vi "SPIM Controller.vi"() -> ()   [LabVIEW 2015]
uses:
  controls/Camera Properties.ctl
  controls/Microscope Settings.ctl
  controls/CameraState.ctl
  controls/ModeEnum.ctl
  controls/PinOut.ctl
  controls/Hardware.ctl
  controls/PinOut2.ctl
  controls/Stack_State.ctl
  controls/Stack Track.ctl
  controls/CameraControlTypeDef.ctl
  <vilib>/DAQmx/create/channels.llb/DAQmx Create Channel (DO-Digital Output).vi
  <vilib>/DAQmx/create/channels.llb/DAQmx Create Channel (AO-Voltage-Basic).vi
  <vilib>/Waveform/DWDTOps.llb/DWDT Append Digital Samples.vi
  <vilib>/Waveform/WDTOps.llb/WDT Append Waveforms DBL.vi
  <vilib>/Waveform/WDTOps.llb/WDT Waveform Duration DBL.vi
  <vilib>/vision/NI_Vision_Development_Module.lvlib
panel:
  out "Numeric 3":i32
  out "Numeric 2":i32
  out "Stack Number":i32
  out "Numeric":i32
  in  "Tab Control":enum32{"Camera Settings", "Recording"}(tab)
  in  "Scan Cont":bool
  in  "Tweezers":T1={"Start /um"=40.0, "Step/um"=5.0, "Range /um"=20.0} {"Range /um" min=0.0 max=10.0 step=0.05; "Step/um" min=0.0001 max=10.0 step=0.05; "Start /um" min=0.0 max=10.0 step=0.05}
  in  "Save to:":path=path "C:/_DATA/test.tiff"
  in  "Scans":dbl=1.0 min=0.0 max=10.0 step=0.05
  in  "?":bool
  in  "Scan":bool
  in  "Scan Continuously":bool
  out "error IO":errorcluster
  in  "Advanced DCAM Controls":i32(listbox) caption="Multicolumn Listbox"
  out "Duration":string
  in  "Microscope Settings":T2={"Mode"=enum."XY", "Slit"={"Scanning Mode"=12.0, "Slit Width /%"=5.0}, "Colour"=[{"Laser"=enum."561", "Filter"=4}], "Exposure/ms"=40.0, "Piezo Position /um"=0.0, "ROI"={"X"={"Start /px"=0.0, "Step /px"=1.0, "Range /px"=2048.0}, "Y"={"Start /px"=0.0, "Step /px"=1.0, "Range /px"=2048.0}, "Z "={"Start /um"=0.0, "Step/um"=1.0, "Range /um"=100.0}, "T "={"Start /s"=0.0, "Step /s"=1.0, "Range /s"=100.0}}, "Samples per millisecond"=100.0, "Relax/ms"=10.0, "Readout Direction"=2.0, "Trigger Source"=2.0, "Camera Delay /ms"=11.0, "Under Scan /ms"=5.0, "Calibration Coordinates"={"Top Left"=[-4.418670520231216, -0.1592138728323702, 10.0], "Top Right"=[-9.501965317919073, -0.1592138728323702, 10.0], "Bottom Left"=[-4.4508670520231215, 0.0, 0.0], "Bottom Right"=[-9.53757225433526, 0.0, 0.0], "Waveforms"={"Analogue Out"=[], "Digital Out"=[]}}} {"Under Scan /ms" min=0.0 max=10.0 step=0.05; "ROI"."T"."Range /s" min=0.0 max=10.0 step=0.05 format="%<%H:%M:%S>t"; "ROI"."T"."Step /s" min=0.0 max=10.0 step=0.05 format="%<%M:%S%2u>t"; "ROI"."T"."Start /s" min=0.0 max=10.0 step=0.05 format="%<%M:%S%2u>t"; "ROI"."X"."Range /px" min=0.0 max=10.0 step=0.05; "ROI"."X"."Step /px" min=0.0 max=10.0 step=0.05; "ROI"."X"."Start /px" min=0.0 max=10.0 step=0.05; "ROI"."Y"."Range /px" min=0.0 max=10.0 step=0.05; "ROI"."Y"."Step /px" min=0.0 max=10.0 step=0.05; "ROI"."Y"."Start /px" min=0.0 max=10.0 step=0.05; "ROI"."Z"."Range /um" min=0.0 max=10.0 step=0.05; "ROI"."Z"."Step/um" min=0.0001 max=10.0 step=0.05; "ROI"."Z"."Start /um" min=0.0 max=10.0 step=0.05; "Colour"."Filter" items=["Empty"=1, ""=2, ""=3, "561"=4, ""=5, "488"=6]; "Camera Delay /ms" min=0.0 max=10.0 step=0.05; "Trigger Source" items=["Internal"=1.0, "External"=2.0]; "Readout Direction" items=["Forward"=1.0, "Backward"=2.0]; "Slit"."Scanning Mode" items=["Full Frame"=1.0, "Slit Scanning"=12.0]; "Piezo Position /um" min=0.0 max=10.0 step=0.05}
  in  "Properties":T3=4211904 items=["SENSOR MODE"=4212128, "CCD MODE"=4212384, "READOUT MODE"=4211872, "ACTIVE VIEW INDEX"=4343136, "BITS PER CHANNEL"=4342976, "IMAGE PIXEL TYPE"=4343296, "BINNING"=4215968, "EXPOSURE TIME"=2049184, "CONTRAST GAIN"=3163312, "CONTRAST OFFSET"=3163328, "LIGHT MODE"=2114720, "SENSITIVITY"=2114992, "PHOTON IMAGING MODE"=2115200, "HIGH DYNAMIC RANGE MODE"=3163360, "WHITE BALANCE"=3163568, "TEMPERATURE"=2115232, "TEMPERATURE TARGET"=2115264, "SENSOR COOLER FAN"=2115296, "LINEBUNDLE HEIGHT"=4212192, "MECHANICAL SHUTTER"=2115488, "BACK FOCUS POSITION"=8422304, "TRIGGER CONNECTOR"=1066432, "TRIGGER SOURCE"=1066144, "OUTPUT TRIGGER SOURCE"=1852576, "TRIGGER GLOBAL EXPOSURE"=2049680, "FIRST TRIGGER BEHAVIOR"=2049696, "CHANNEL SYNC"=1852352, "READOUT DIRECTION"=4211904, "PRE HSYNC COUNT"=1852704, "INTERNAL LINE SPEED"=4191408, "INTERNAL LINE INVERVAL"=4191424]
  out "Enum":T4=enum."active"
  out "FPS":dbl
  in  "Multicolumn Listbox":i32(listbox)
  out "Image":T5(plugin-control)
  out "Histogram":T6(graph)
  in  "stop":bool
  in  "Load Settings":bool
  in  "Save Settings":bool
  in  "Frames":i32
  in  "Record":bool
  in  "Signals Debugger":bool
  in  "Stage Controller":bool
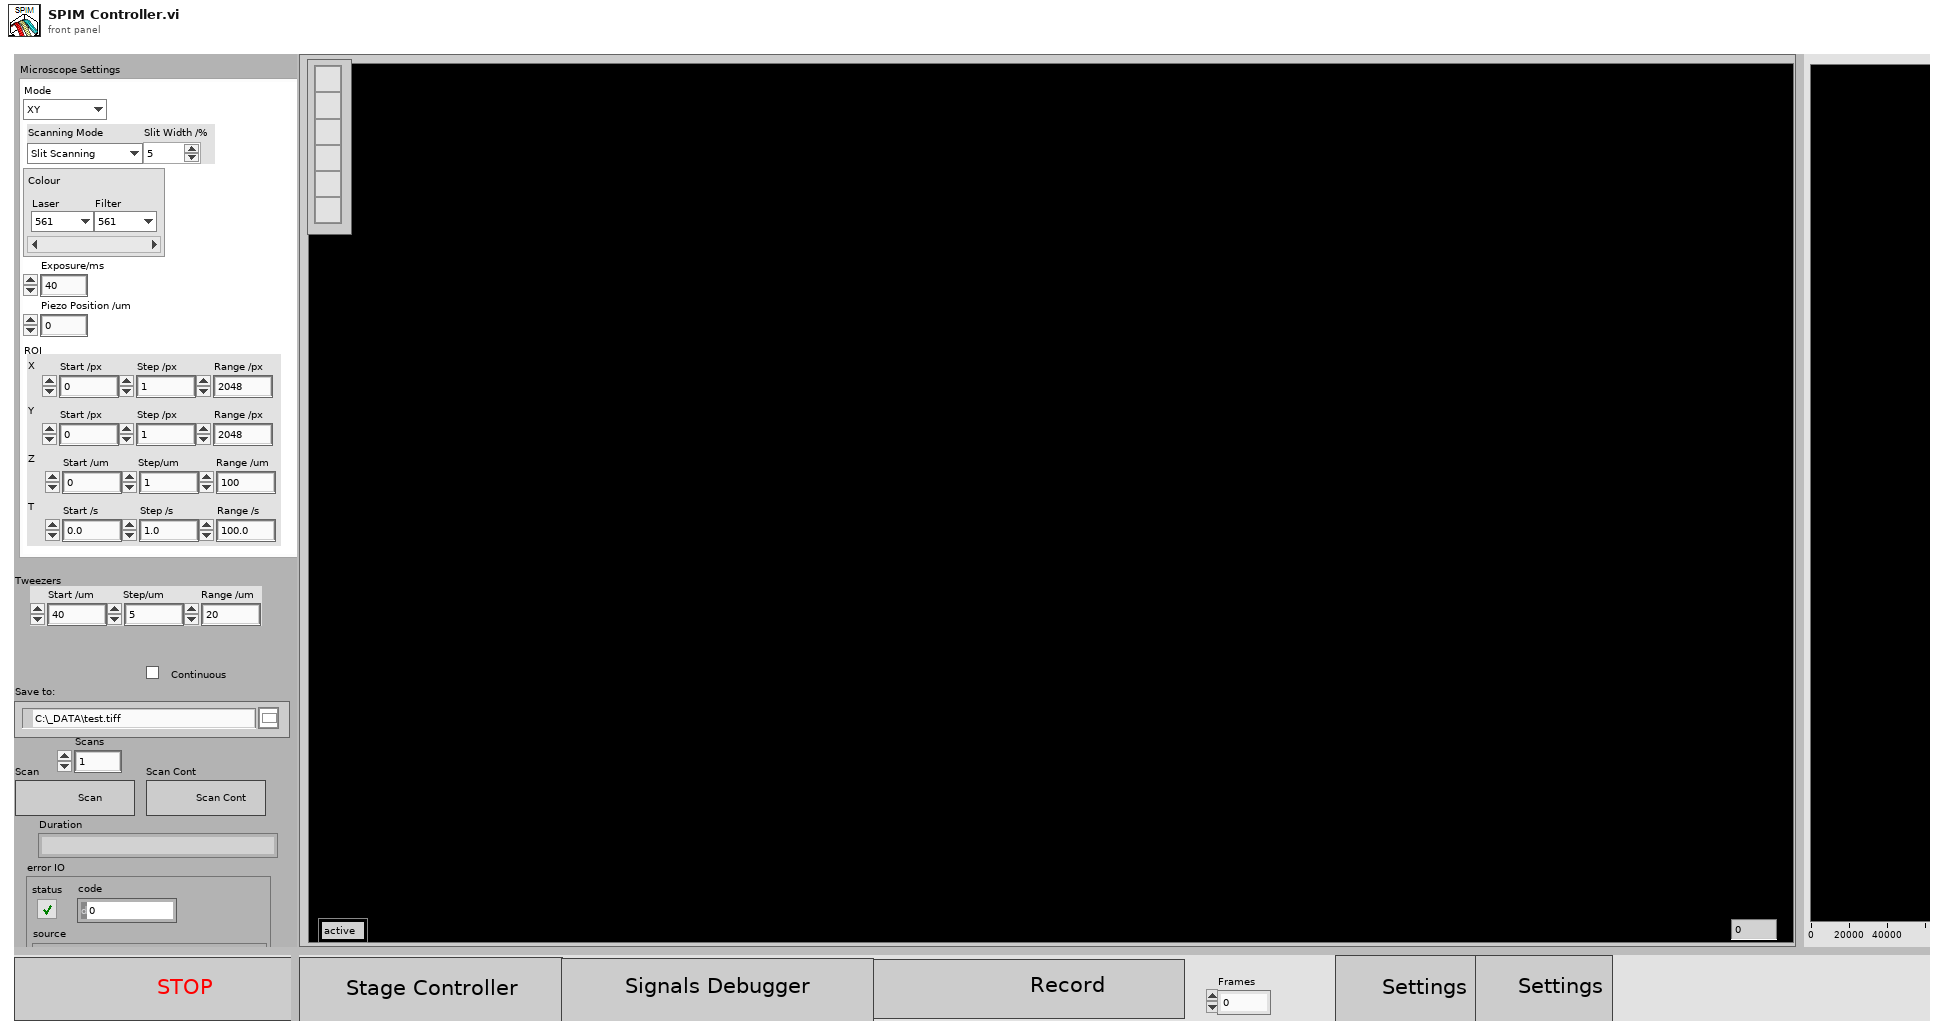
[diagram p1: front panel]
types:
  T1 = cluster{"Start /um":dbl, "Step/um":dbl, "Range /um":dbl}
  T2 = typedef "Microscope Settings.ctl" = cluster{"Mode":enum16{"X", "XY", "XYZ", "XYZT", "XYZC", "Tweezers", "Virus"}, "Slit":cluster{"Scanning Mode":dbl, "Slit Width /%":dbl}, "Colour":cluster{"Laser":enum16{"Brightfield", "445", "488", "561", "647"}, "Filter":u16}[], "Exposure/ms":dbl, "Piezo Position /um":dbl, "ROI":cluster{"X":cluster{"Start /px":dbl, "Step /px":dbl, "Range /px":dbl}, "Y":cluster{"Start /px":dbl, "Step /px":dbl, "Range /px":dbl}, "Z ":cluster{"Start /um":dbl, "Step/um":dbl, "Range /um":dbl}, "T ":cluster{"Start /s":dbl, "Step /s":dbl, "Range /s":dbl}}, "Samples per millisecond":dbl, "Relax/ms":dbl, "Readout Direction":dbl, "Trigger Source":dbl, "Camera Delay /ms":dbl, "Under Scan /ms":dbl, "Calibration Coordinates":cluster{"Top Left":dbl[], "Top Right":dbl[], "Bottom Left":dbl[], "Bottom Right":dbl[], "Waveforms":cluster{"Analogue Out":waveform(dbl)[], "Digital Out":digitalwaveform[]}}}
  T3 = typedef "Camera Properties.ctl" = u32
  T4 = typedef "CameraState.ctl" = enum16{"init", "active", "deinit"}
  T5 = typedef "IMAQ Image.ctl" = refnum<image>
  T6 = cluster{"Starting Value":sgl, "Incremental Value":sgl, "Histogram":u32[]}
  T7 = cluster{"height":u32, "width":u32, "datatype":u32}
  T8 = typedef "Hardware.ctl" = enum16{"Stop", "RunCont", "EndCont", "Idle", "Update", "Run Waves"}
  T9 = typedef "PinOut.ctl" = string
  T10 = typedef "ModeEnum.ctl" = enum16{"Idle", "generateWaves", "runWaves", "runWavesCont", "endWavesCont", "stop"}
  T11 = cluster{"Mode":u32, "Polarity":u32, "Times":u32, "Delay":dbl}
  T12 = typedef "Stack_State.ctl" = cluster{"State":T13, "Stack Number":i32, "Image":u16[][], "Stacks":i32}
  T13 = typedef "Stack Track.ctl" = enum16{"Idle", "Display", "Start Sequence", "Read Disk", "STOP", "Collecting", "End", "Save Image"}
  T14 = typedef "CameraControlTypeDef.ctl" = enum16{"Idle", "IntervalLineInt", "Ram Record", "HardDisk Record", "Disengage Update", "Update", "ROI", "Binning", "Scan Mode", "Trigger Mode", "Readout Mode", "Readout Direction", "Preview", "ROIWindow", "Trigger Source"}
  T15 = cluster{"Laser":enum16{"Brightfield", "445", "488", "561", "647"}, "Filter":u16}[]
  T16 = enum32{"Invalid", "Standard", "Closed", "Hidden", "Minimized", "Maximized"}
  T17 = enum16{"open", "replace", "create", "open or create", "replace or create", "replace or create with confirmation"}
  T18 = typedef "PinOut2.ctl" = string
  T19 = cluster{"Analogue Out":waveform(dbl)[], "Digital Out":digitalwaveform[]}
  T20 = enum16{"X", "XY", "XYZ", "XYZT", "XYZC", "Tweezers", "Virus"}
  T21 = typedef "Image Type" = u32
  T22 = cluster{"Analogue Out out":waveform(dbl)[], "Digital Out out":digitalwaveform[]}
  T23 = cluster{"State":T13, "Timeout":i32, "Data 16":u16[][], "Timeout":i32}
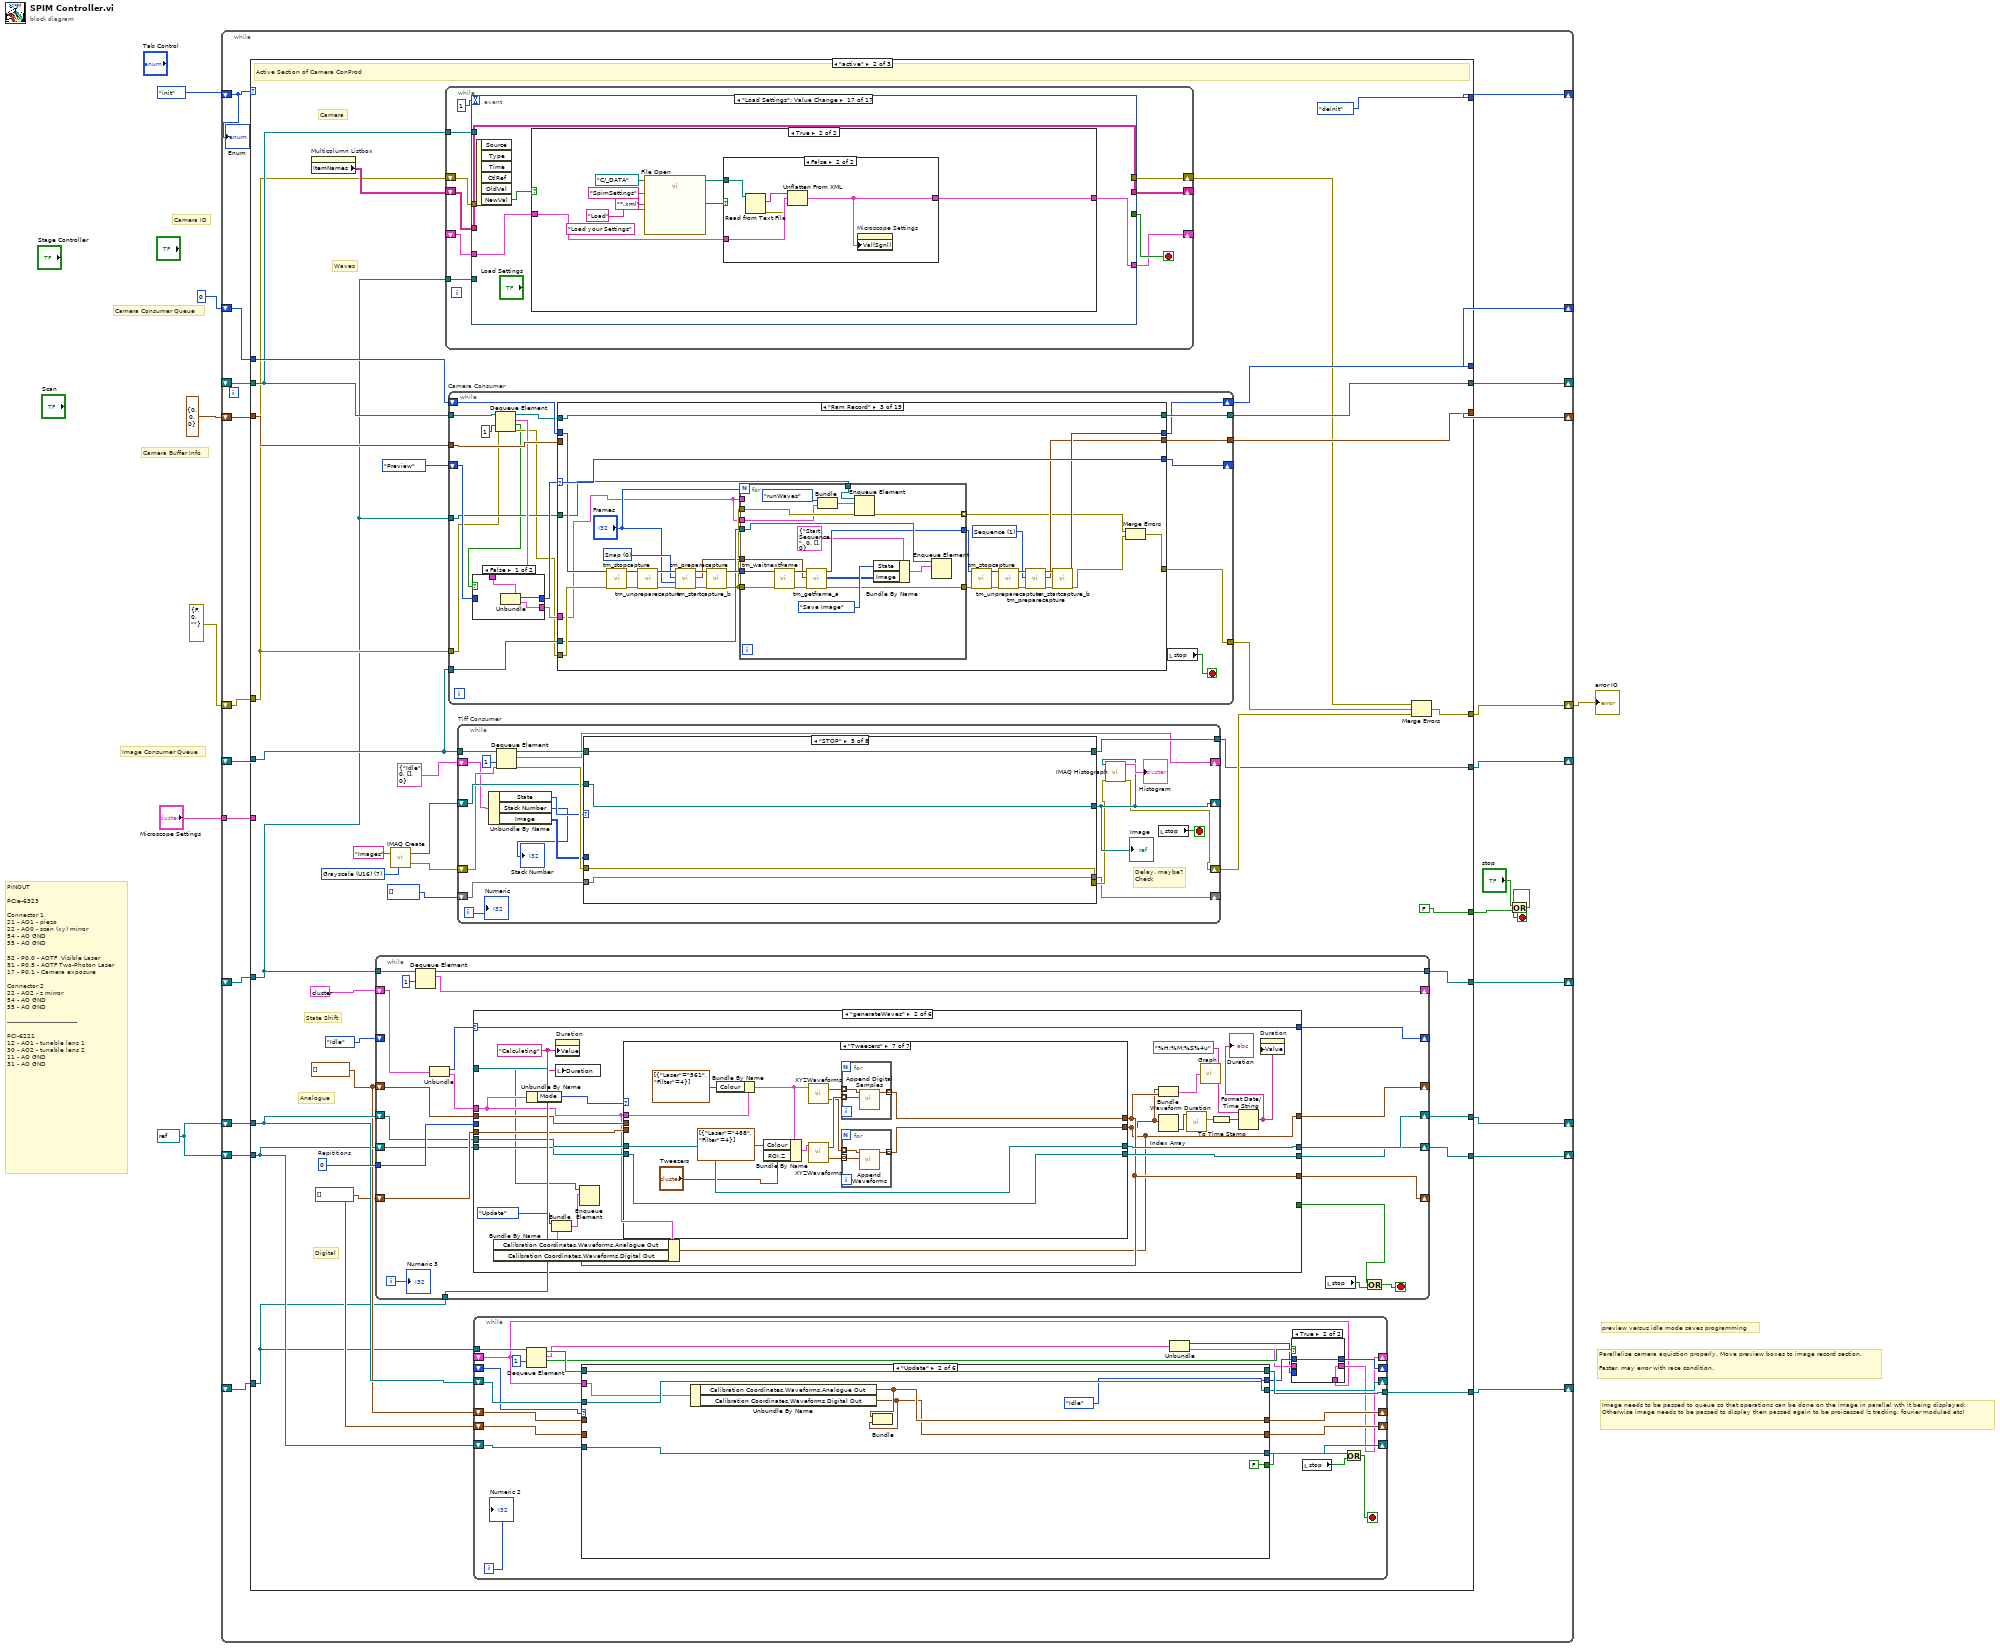
[diagram p0: block diagram]
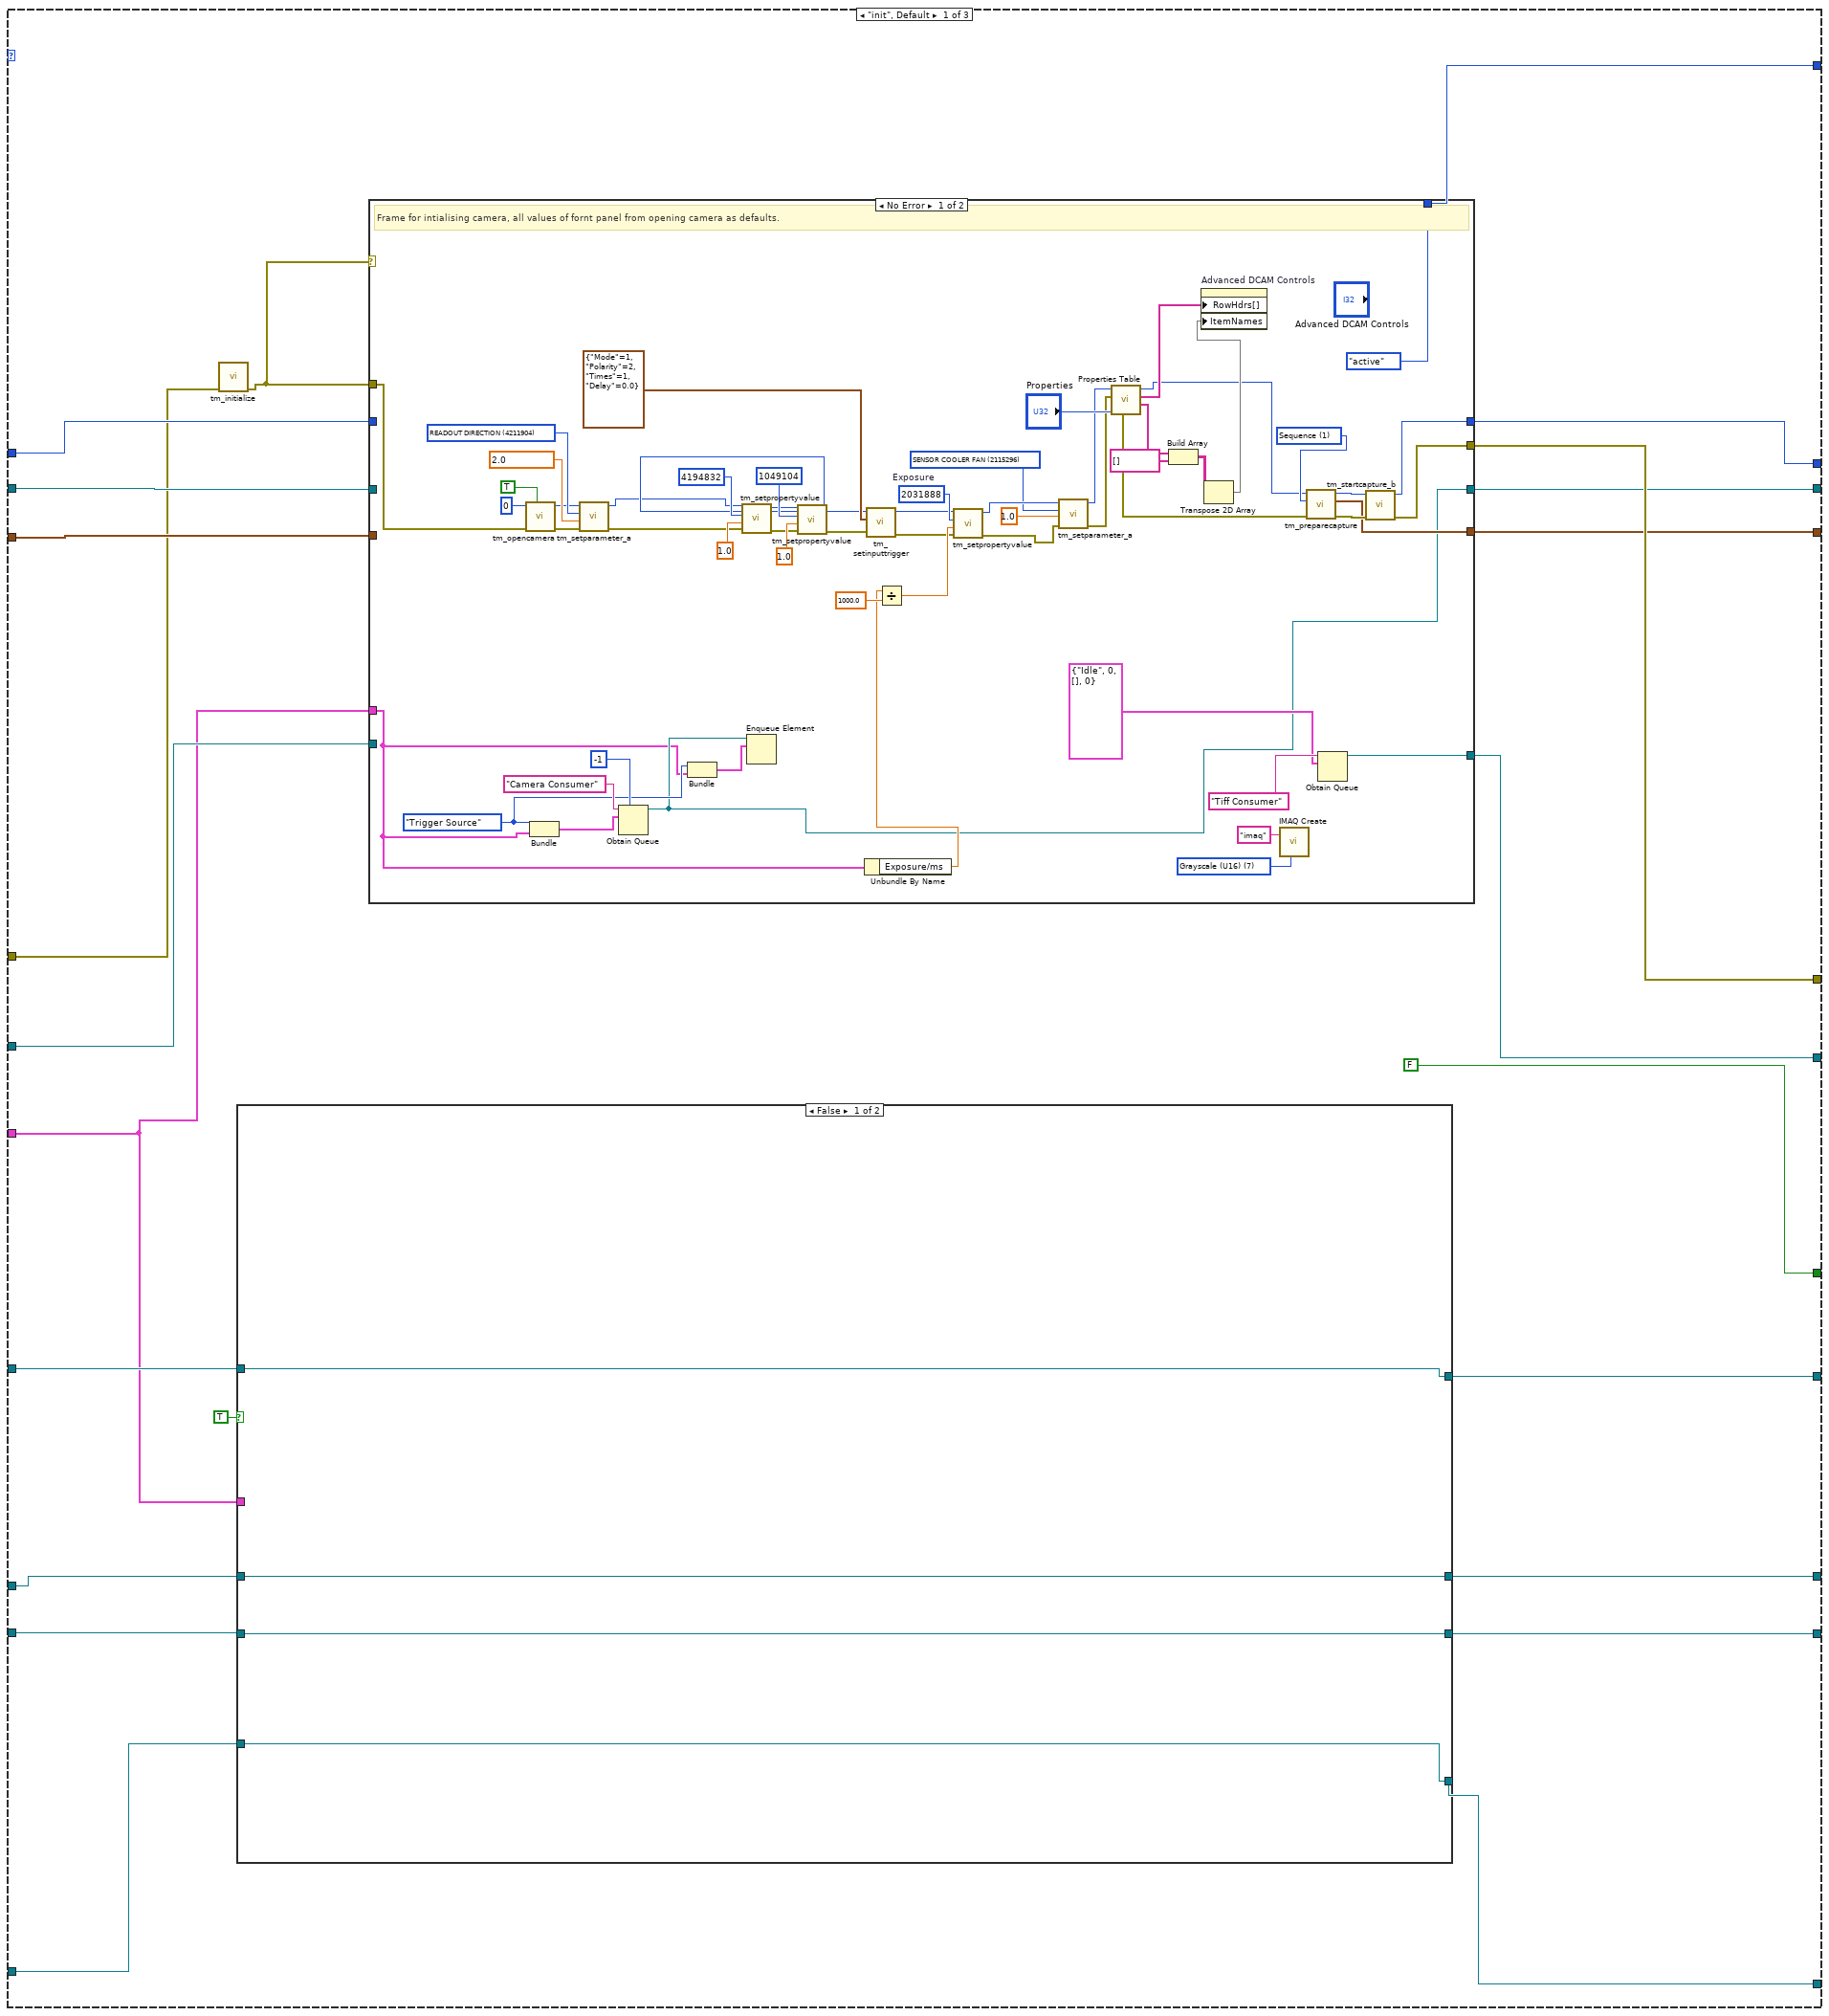
[diagram p2: hidden frame]
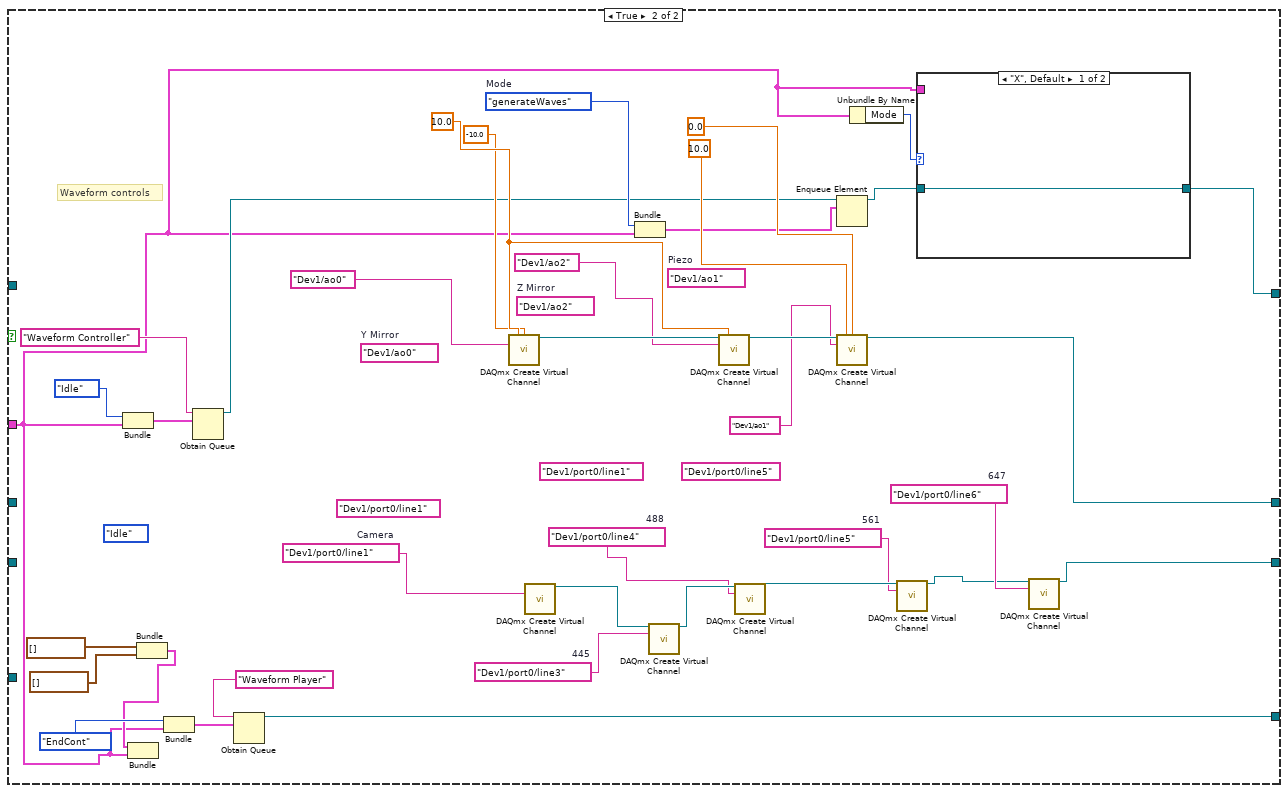
[diagram p3: hidden frame]
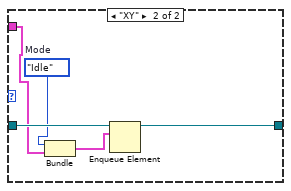
[diagram p4: hidden frame]
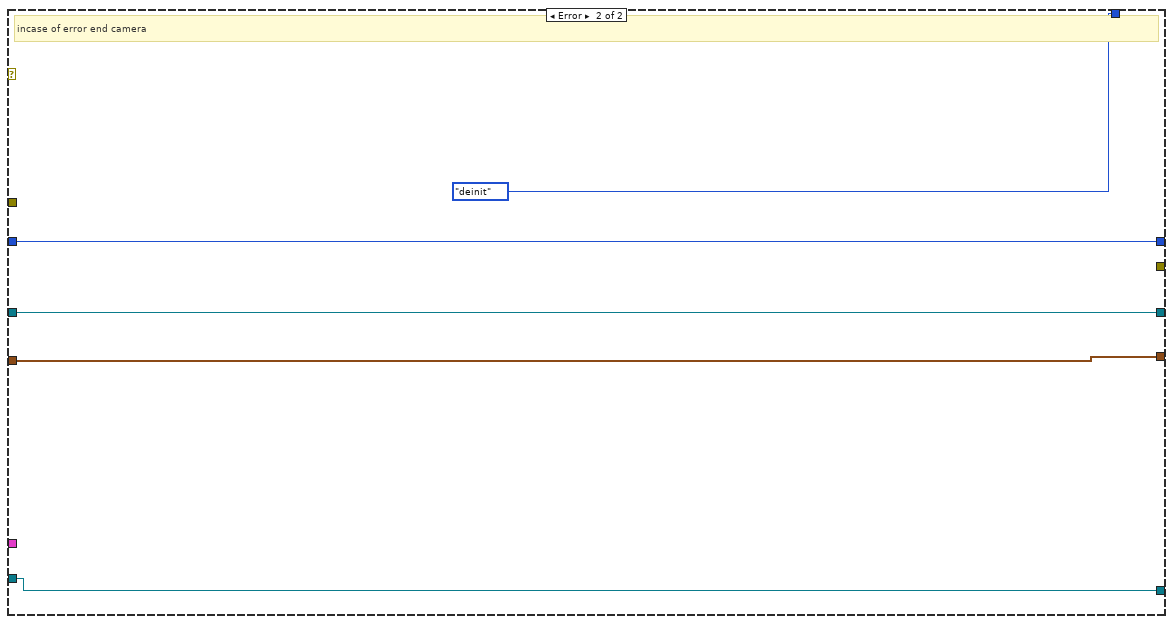
[diagram p5: hidden frame]
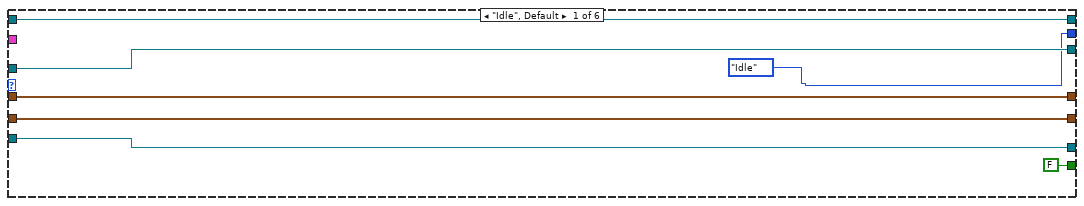
[diagram p7: hidden frame]
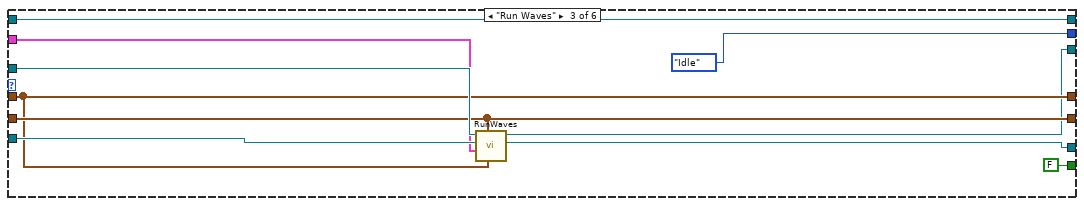
[diagram p8: hidden frame]
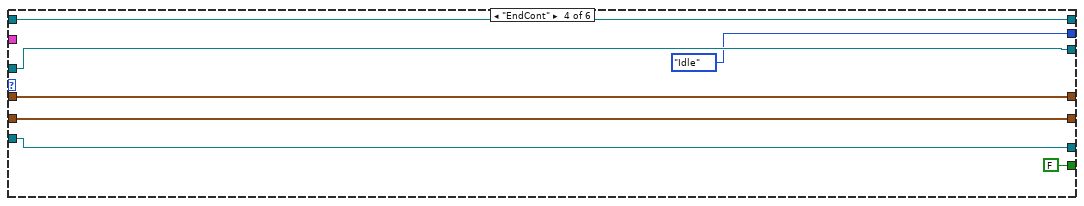
[diagram p9: hidden frame]
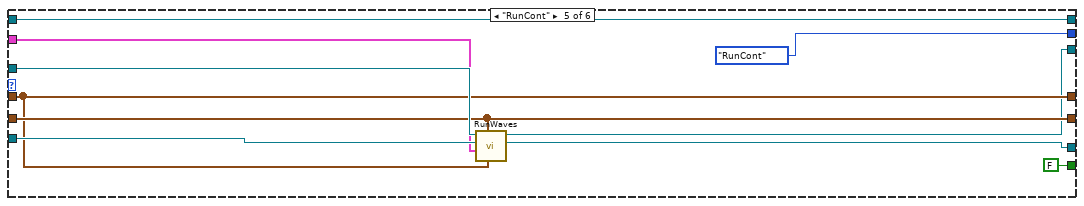
[diagram p10: hidden frame]
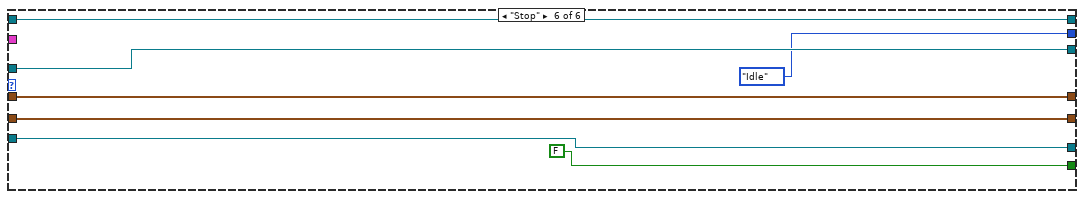
[diagram p11: hidden frame]
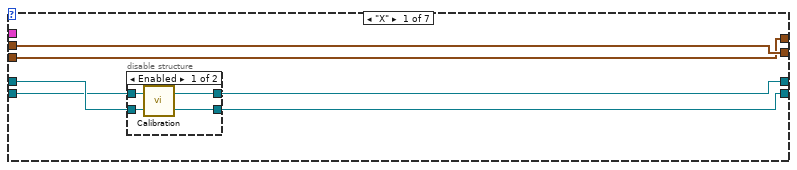
[diagram p13: hidden frame]
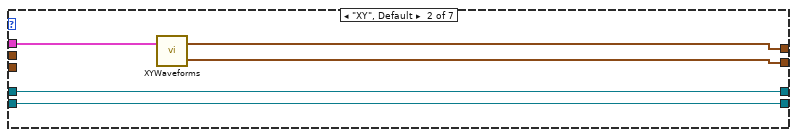
[diagram p15: hidden frame]
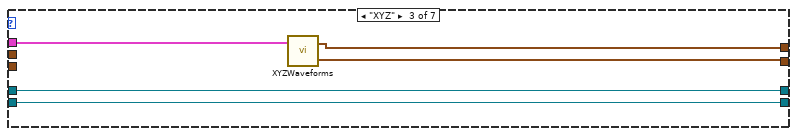
[diagram p16: hidden frame]
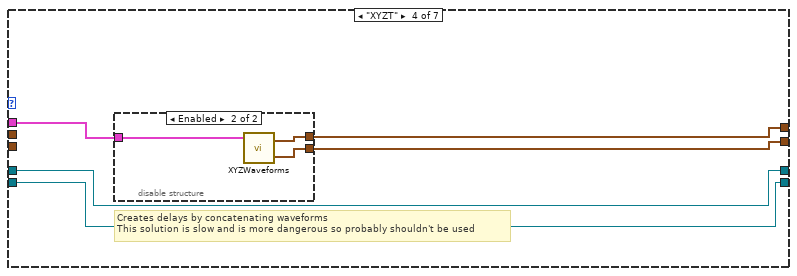
[diagram p17: hidden frame]
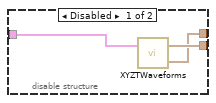
[diagram p18: hidden frame]
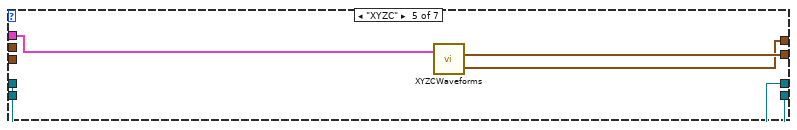
[diagram p19: hidden frame]
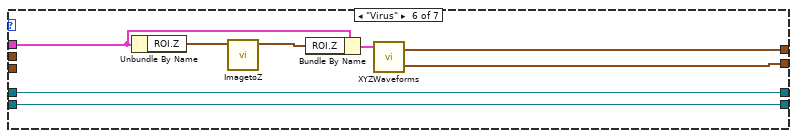
[diagram p20: hidden frame]
diagram:
  w4 = refnum<k21> refnum ("Mirror Z 2")
  # "PINOUT\n\nPCIe-6323\n\nConnector 1\n21 - AO1 - piezo\n22 - AO0 - scan (xy) mirror\n54 - AO GND\n55 - AO GND\n\n52 - P0.0 - AOTF  Visible Laser\n51 - P0.5 - AOTF Two-Photon Laser\n17 - P0.1 - Camera exposure\n\nConnector 2\n22 - AO2 - z mirror\n54 - AO GND\n55 - AO GND\n\n-----------------------------------\n\nPCI-6221\n12 - AO1 - tunable lens 1\n30 - AO2 - tunable lens 2\n11 - AO GND\n31 - AO GND"
  # "Camera Buffer Info"
  # "Image needs to be passed to queue so that operations can be done on the image in parallel wth it being displayed;\nOtherwise image needs to be passed to display then passed again to be proicessed (z tracking, fourier moduled etc)"
  # "preview versus idle mode saves programming"
  # "Parallelise camera aquistion properly. Move preview boxes to image record section.\n\nFaster. may error with race condition."
  # "Image Consumer Queue"
  # "Camera Consumer Queue"
  # "Camera ID"
  n1 = while {
    shift-right: [w31] -> _
    shift-left: CameraState."init" -> [w9]
    shift-right: [w30] -> _
    shift-left: u32 0 ("Handle out") -> [w29]
    shift-right: [w28] -> w6
    shift-left: errorcluster {"status"=FALSE, "code"=0, "source"=""} ("error IO") -> [w27]
    shift-right: [w26] -> _
    shift-left: _ -> [w25]
    shift-right: [w12] -> _
    shift-left: _ -> [w24]
    shift-right: [w20] -> _
    shift-left: T7 {"height"=0, "width"=0, "datatype"=0} ("Buffer Info") -> [w19]
    shift-right: [w18] -> _
    shift-left: w4 -> [w17]
    shift-right: [w15] -> _
    shift-left: w4 -> [w16]
    shift-right: [w14] -> _
    shift-left: _ -> [w13]
    shift-right: [w11] -> _
    shift-left: _ -> [w10]
    tunnel: "Microscope Settings" -> [w8]
    stop <- w22 stop-if-true
    n2 = case shown="\"active\"" w9 {
      tunnel: [w54 CameraState."deinit" CameraState."init"] -> w31
      tunnel: [w53 w198 w959] -> w30
      tunnel: w29 -> [w43 w199 w959]
      tunnel: [w52 w197 w962] -> w28
      tunnel: w27 -> [w41 w179 w963]
      tunnel: [w51 w194 w947] -> w12
      tunnel: [w50 w193 w943] -> w26
      tunnel: w25 -> [w48 w187 w943]
      tunnel: w24 -> [w49 w186 w947]
      tunnel: [FALSE ("stop") FALSE ("stop") TRUE ("stop")] -> w21
      tunnel: [w46 w190 w956] -> w20
      tunnel: w19 -> [w45 w189 w956]
      tunnel: w13 -> [w38 w173 w942]
      tunnel: [w44 w183 w954] -> w18
      tunnel: w17 -> [w37 w172 w954]
      tunnel: w16 -> [w36 w171 w952]
      tunnel: [w42 w184 w952] -> w15
      tunnel: [w39 w182 w942] -> w14
      tunnel: [w34 w168 w941] -> w11
      tunnel: w10 -> [w33 w167 w941]
      tunnel: w8 -> [w32 _ _]
      frame "init", Default {
        n3 = call "tm_initialize.vi"("error in (no error)"=w41) -> ("error out"=w40:errorcluster)  [unwired: 7 in, 3 out]
        n4 = case shown="False" TRUE {
          tunnel: [w57 w91] -> w44
          tunnel: [w56 w67] -> w42
          tunnel: w32 -> [_ w59]
          tunnel: [w58 w80] -> w39
          tunnel: w38 -> [w58 _]
          tunnel: w37 -> [w57 _]
          tunnel: w36 -> [w56 _]
          tunnel: [w55 w62] -> w34
          tunnel: w33 -> [w55 _]
          frame False {
          }
          frame True {
            (unwired) ModeEnum."Idle" ("Mode")
            w69 = tag "Dev1/port0/line6"  # 647
            w71 = tag "Dev1/port0/line5"  # 561
            w76 = tag "Dev1/port0/line3"  # 445
            (unwired) T9 "Dev1/port0/line1" ("Combo Box")
            (unwired) T18 "Dev1/port0/line1" ("Combo Box")
            (unwired) T9 "Dev1/port0/line5" ("Combo Box")
            w73 = tag "Dev1/port0/line4"  # 488
            w70 = tag "Dev1/port0/line1"  # Camera
            w88 = ModeEnum."generateWaves"  # Mode
            (unwired) tag "Dev1/ao1"  # Piezo
            (unwired) tag "Dev1/ao2"  # Z Mirror
            (unwired) tag "Dev1/ao0"  # Y Mirror
            w95 = 10.0 ("maximum value")
            # "Waveform controls"
            n5 = Bundle("Mode"=ModeEnum."Idle", "Microscope Settings"=w59) -> (w86:cluster{"Mode":T10, "Microscope Settings":T2})  [unwired: 1 in]
            n6 = Bundle "Bundle"("Analogue Out"=waveform(dbl)[] [], "Digital Out"=digitalwaveform[] []) -> (w60:T19)  [unwired: 1 in]
            n7 = Bundle(w60, "Microscope Settings"=w59) -> ()  [unwired: 1 in, 1 out]
            n8 = Bundle(Hardware."EndCont", "Microscope Settings"=w59) -> (w66:cluster{T8, "Microscope Settings":T2})  [unwired: 1 in]
            n9 = Obtain Queue(name (unnamed)="Waveform Controller", element data type=w86) -> (queue out=w85:refnum<queue>)  [unwired: 3 in, 2 out]
            n10 = Obtain Queue(name (unnamed)="Waveform Player", element data type=w66) -> (queue out=w62:refnum<queue>)  [unwired: 3 in, 2 out]
            n11 = call-poly <vilib>:"DAQmx Create Virtual Channel.vi"("maximum value"=w95, "minimum value"=-10.0, "physical channels"=T9 "Dev1/ao0" ("Combo Box")) -> ("task out"=w90:refnum<k21>)  [unwired: 11 in, 1 out]
            n12 = call-poly <vilib>:"DAQmx Create Virtual Channel.vi"("lines"=w70) -> ("task out"=w75:refnum<k21>)  [unwired: 13 in, 1 out]
            n13 = Bundle("Mode"=w88, "Microscope Settings"=w59) -> (w82:cluster{"Mode":T10, "Microscope Settings":T2})  [unwired: 1 in]
            n14 = call-poly <vilib>:"DAQmx Create Virtual Channel.vi"("task in"=w75, "lines"=w76) -> ("task out"=w74:refnum<k21>)  [unwired: 12 in, 1 out]
            n15 = call-poly <vilib>:"DAQmx Create Virtual Channel.vi"("task in"=w90, "maximum value"=w95, "physical channels"=T9 "Dev1/ao2" ("Combo Box")) -> ("task out"=w89:refnum<k21>)  [unwired: 11 in, 1 out]
            n16 = call-poly <vilib>:"DAQmx Create Virtual Channel.vi"("task in"=w74, "lines"=w73) -> ("task out"=w72:refnum<k21>)  [unwired: 12 in, 1 out]
            n17 = Enqueue Element(queue=w85, element=w82) -> (queue out=w83:refnum<queue>)  [unwired: 2 in, 2 out]
            n18 = call-poly <vilib>:"DAQmx Create Virtual Channel.vi"("task in"=w89, "maximum value"=10.0 ("minimum value"), "minimum value"=0.0 ("maximum value"), "physical channels"=T9 "Dev1/ao1" ("Combo Box")) -> ("task out"=w91:refnum<k21>)  [unwired: 10 in, 1 out]
            n19 = Unbundle By Name(w59) -> ("Mode"=w81:T20)
            n20 = call-poly <vilib>:"DAQmx Create Virtual Channel.vi"("task in"=w72, "lines"=w71) -> ("task out"=w68:refnum<k21>)  [unwired: 12 in, 1 out]
            n21 = case shown="\"X\", Default" w81 {
              tunnel: w83 -> [w96 w101]
              tunnel: w59 -> [_ w99]
              tunnel: [w96 w97] -> w80
              frame "X", Default {
              }
              frame "XY" {
                w98 = ModeEnum."Idle"  # Mode
                n22 = Bundle("Mode"=w98, "Microscope Settings"=w99) -> (w100:cluster{"Mode":T10, "Microscope Settings":T2})  [unwired: 1 in]
                n23 = Enqueue Element(queue=w101, element=w100) -> (queue out=w97:refnum<queue>)  [unwired: 2 in, 2 out]
              }
            }
            n24 = call-poly <vilib>:"DAQmx Create Virtual Channel.vi"("task in"=w68, "lines"=w69) -> ("task out"=w67:refnum<k21>)  [unwired: 12 in, 1 out]
          }
        }
        n25 = case shown="No Error" w40 {
          tunnel: w40 -> [w127 _]
          tunnel: [CameraState."active" CameraState."deinit"] -> w54
          tunnel: [w154 _] -> w52
          tunnel: [w152 w159] -> w53
          tunnel: [w104 w162] -> w51
          tunnel: [w149 w161] -> w50
          tunnel: w49 -> [_ w162]
          tunnel: w48 -> [_ w161]
          tunnel: [w147 w160] -> w46
          tunnel: w45 -> [_ w160]
          tunnel: w43 -> [_ w159]
          tunnel: w32 -> [w103 _]
          frame No Error {
            w124 = u32 2115296 items=["SENSOR MODE"=4212128, "CCD MODE"=4212384, "READOUT MODE"=4211872, "ACTIVE VIEW INDEX"=4343136, "BITS PER CHANNEL"=4342976, "IMAGE PIXEL TYPE"=4343296, "BINNING"=4215968, "EXPOSURE TIME"=2049184, "CONTRAST GAIN"=3163312, "CONTRAST OFFSET"=3163328, "LIGHT MODE"=2114720, "SENSITIVITY"=2114992, "PHOTON IMAGING MODE"=2115200, "HIGH DYNAMIC RANGE MODE"=3163360, "WHITE BALANCE"=3163568, "TEMPERATURE"=2115232, "TEMPERATURE TARGET"=2115264, "SENSOR COOLER FAN"=2115296, "LINEBUNDLE HEIGHT"=4212192, "MECHANICAL SHUTTER"=2115488, "BACK FOCUS POSITION"=8422304, "TRIGGER CONNECTOR"=1066432, "TRIGGER SOURCE"=1066144, "OUTPUT TRIGGER SOURCE"=1852576, "TRIGGER GLOBAL EXPOSURE"=2049680, "FIRST TRIGGER BEHAVIOR"=2049696, "CHANNEL SYNC"=1852352, "READOUT DIRECTION"=4211904, "PRE HSYNC COUNT"=1852704, "INTERNAL LINE SPEED"=4226000, "INTERNAL LINE INTERVAL"=4226016] ("Parameter")
            w106 = CameraControlTypeDef."Trigger Source" ("Enum")
            w131 = u32 2031888  # Exposure
            w142 = sgl 2.0 items=["Forward"=1.0, "Backward"=2.0] ("Readout Direction")
            w143 = u32 4211904 items=["SENSOR MODE"=4212128, "CCD MODE"=4212384, "READOUT MODE"=4211872, "ACTIVE VIEW INDEX"=4343136, "BITS PER CHANNEL"=4342976, "IMAGE PIXEL TYPE"=4343296, "BINNING"=4215968, "EXPOSURE TIME"=2049184, "CONTRAST GAIN"=3163312, "CONTRAST OFFSET"=3163328, "LIGHT MODE"=2114720, "SENSITIVITY"=2114992, "PHOTON IMAGING MODE"=2115200, "HIGH DYNAMIC RANGE MODE"=3163360, "WHITE BALANCE"=3163568, "TEMPERATURE"=2115232, "TEMPERATURE TARGET"=2115264, "SENSOR COOLER FAN"=2115296, "LINEBUNDLE HEIGHT"=4212192, "MECHANICAL SHUTTER"=2115488, "BACK FOCUS POSITION"=8422304, "TRIGGER CONNECTOR"=1066432, "TRIGGER SOURCE"=1066144, "OUTPUT TRIGGER SOURCE"=1852576, "TRIGGER GLOBAL EXPOSURE"=2049680, "FIRST TRIGGER BEHAVIOR"=2049696, "CHANNEL SYNC"=1852352, "READOUT DIRECTION"=4211904, "PRE HSYNC COUNT"=1852704, "INTERNAL LINE SPEED"=4226000, "INTERNAL LINE INTERVAL"=4226016] ("Parameter")
            w146 = T21 7 items=["Grayscale (U8)", "Grayscale (I16)", "Grayscale (SGL)", "Complex (CSG)", "RGB (U32)", "HSL (U32)", "RGB (U64)", "Grayscale (U16)"] ("Image Type")
            w156 = 1 items=["Snap", "Sequence"] ("Capture mode")
            # "Frame for intialising camera, all values of fornt panel from opening camera as defaults."
            n26 = call "tm_opencamera.vi"("Force Open"=TRUE, "error in (no error)"=w127, "Camera Index"=u32 0) -> ("error out"=w140:errorcluster, "Handle out"=w141:u32)  [unwired: 6 in, 1 out]
            n27 = Bundle("Enum"=w106, "Microscope Settings"=w103) -> (w105:cluster{"Enum":T14, "Microscope Settings":T2})  [unwired: 1 in]
            n28 = call "tm_setparameter_a.vi"("error in (no error)"=w140, "Value in"=w142, "Parameter"=w143, "Handle in"=w141) -> ("error out"=w113:errorcluster, "Handle out"=w132:u32)  [unwired: 6 in]
            n29 = Obtain Queue(max queue size (-1, unlimited)=-1, name (unnamed)="Camera Consumer", element data type=w105) -> (queue out=w104:refnum<queue>)  [unwired: 2 in, 2 out]
            n30 = Bundle("Enum"=w106, "Microscope Settings"=w103) -> (w102:cluster{"Enum":T14, "Microscope Settings":T2})  [unwired: 1 in]
            n31 = call "tm_setpropertyvalue.vi"("error in (no error)"=w113, "Value in"=sgl 1.0, "Property ID"=u32 4194832, "Handle in"=w132) -> ("error out"=w112:errorcluster, "Handle out"=w135:u32)  [unwired: 6 in]
            n32 = Enqueue Element(queue=w104, element=w102) -> ()  [unwired: 2 in, 3 out]
            n33 = call "tm_setpropertyvalue.vi"("error in (no error)"=w112, "Value in"=sgl 1.0, "Property ID"=u32 1049104, "Handle in"=w135) -> ("error out"=w111:errorcluster, "Handle out"=w133:u32)  [unwired: 6 in]
            n34 = Unbundle By Name(w103) -> ("Exposure/ms"=w114:dbl)
            n35 = call "tm_setinputtrigger.vi"("error in (no error)"=w111, "Parameters"=T11 {"Mode"=1, "Polarity"=2, "Times"=1, "Delay"=0.0}, "Handle in"=w133) -> ("error out"=w110:errorcluster, "Handle out"=w130:u32)  [unwired: 7 in]
            n36 = Divide(x=w114, y=sgl 1000.0) -> (x/y=w128:dbl)
            n37 = call "tm_setpropertyvalue.vi"("error in (no error)"=w110, "Value in"=w128, "Property ID"=w131, "Handle in"=w130) -> ("error out"=w109:errorcluster, "Handle out"=w125:u32)  [unwired: 6 in]
            n38 = call "tm_setparameter_a.vi"("error in (no error)"=w109, "Value in"=1.0, "Parameter"=w124, "Handle in"=w125) -> ("error out"=w107:errorcluster, "Handle out"=w116:u32)  [unwired: 6 in]
            n39 = call "Properties Table.vi"("Properties"="Properties", "error in (no error)"=w107, "Handle In"=w116) -> ("Value Stirngs Out"=w120:string[], "Row Headers"=w121:string[], "Handle Out"=w115:u32, "error out"=w108:errorcluster)  [unwired: 1 in, 1 out]
            n40 = Build Array(w120, string[] [] ("element")) -> (w118:string[][])
            n41 = Transpose 2D Array(2D array=w118) -> (transposed array=w117:string[][])
            n42 = property on="Advanced DCAM Controls" class="MCListbox (strict)"("RowHdrs[]"=w121, "ItemNames"=w117) -> ()  [unwired: 2 in, 2 out]
            n43 = call "IMAQ Create"("Image Name"="imaq", "Image Type"=w146) -> ()  [unwired: 3 in, 2 out]
            n44 = call "tm_preparecapture.vi"("error in (no error)"=w108, "Capture mode"=w156, "Handle in"=w115) -> ("error out"=w155:errorcluster, "Buffer Info"=w147:T7, "Handle out"=w153:u32)  [unwired: 5 in, 1 out]
            n45 = Obtain Queue(name (unnamed)="Tiff Consumer", element data type=T12 {"State"=enum."Idle", "Stack Number"=0, "Image"=[], "Stacks"=0} ("input cluster")) -> (queue out=w149:refnum<queue>)  [unwired: 3 in, 2 out]
            n46 = call "tm_startcapture_b.vi"("error in (no error)"=w155, "Handle in"=w153) -> ("error out"=w154:errorcluster, "Handle out"=w152:u32)  [unwired: 8 in]
          }
          frame Error {
            # "incase of error end camera"
          }
        }
      }
      frame "active" {
        w166 = T21 7 items=["Grayscale (U8)", "Grayscale (I16)", "Grayscale (SGL)", "Complex (CSG)", "RGB (U32)", "HSL (U32)", "RGB (U64)", "Grayscale (U16)"] ("Image Type")
        w169 = digitalwaveform[] [] ("Digital Out")
        w170 = waveform(dbl)[] [] ("Analogue Out")
        w185 = 0  # Repititions
        # "State Shift"
        # "Waves"
        # "Camera"
        # "Digital"
        # "Analogue"
        # "Active Section of Camera ConProd"
        n47 = property on="Multicolumn Listbox" class="MCListbox (strict)"() -> ("ItemNames"=w181:string[][])  [unwired: 2 in, 2 out]
        n48 = while {
          tunnel: w173 -> [w299]
          shift-right: [w298] -> _
          shift-left: w170 -> [w297]
          tunnel: w185 -> [w296]
          shift-right: [w292] -> w183
          shift-left: w172 -> [w291]
          shift-right: [w295] -> _
          shift-left: w169 -> [w294]
          shift-right: [w290] -> w184
          shift-left: w171 -> [w289]
          tunnel: [w288] -> w182
          shift-right: [w284] -> _
          shift-left: ModeEnum."Idle" ("Mode") -> [_]
          tunnel: w167 -> [w281]
          shift-right: [w279] -> _
          shift-left: cluster{"Mode":T10, "Microscope Settings":T2} {"Mode"=enum."Idle", "Microscope Settings"={"Mode"=enum."X", "Slit"={"Scanning Mode"=0.0, "Slit Width /%"=0.0}, "Colour"=[], "Exposure/ms"=0.0, "Piezo Position /um"=0.0, "ROI"={"X"={"Start /px"=0.0, "Step /px"=0.0, "Range /px"=0.0}, "Y"={"Start /px"=0.0, "Step /px"=0.0, "Range /px"=0.0}, "Z "={"Start /um"=0.0, "Step/um"=0.0, "Range /um"=0.0}, "T "={"Start /s"=0.0, "Step /s"=0.0, "Range /s"=0.0}}, "Samples per millisecond"=0.0, "Relax/ms"=0.0, "Readout Direction"=0.0, "Trigger Source"=0.0, "Camera Delay /ms"=0.0, "Under Scan /ms"=0.0, "Calibration Coordinates"={"Top Left"=[], "Top Right"=[], "Bottom Left"=[], "Bottom Right"=[], "Waveforms"={"Analogue Out"=[], "Digital Out"=[]}}}} -> [w278]
          i -> [w280]
          stop <- w285 stop-if-true
          n49 = Dequeue Element(queue=w299, timeout in ms (-1)=1) -> (queue out=w288:refnum<queue>, element=w279:cluster{"Mode":T10, "Microscope Settings":T2})  [unwired: 1 in, 2 out]
          n50 = Unbundle(w278) -> ("Mode"=w283:T10, "Microscope Settings"=w282:T2)
          n51 = case shown="\"generateWaves\"" w283 {
            selector: w283 -> [w300 w313 w399 w408 w417 w420]
            tunnel: [_ _ _ _ _ TRUE] -> w287
            tunnel: w282 -> [_ w312 w395 w404 w413 _]
            tunnel: [w304 w308 w397 w406 w415 w425] -> w298
            tunnel: w297 -> [w304 w324 w397 w406 w415 w425]
            tunnel: w296 -> [_ _ _ _ _ _]
            tunnel: [w301 w314 w401 w410 w419 w424] -> w290
            tunnel: [w302 w316 w400 w409 w418 w423] -> w292
            tunnel: w291 -> [w302 w317 w400 w409 w418 w423]
            tunnel: [w303 w309 w396 w405 w414 w422] -> w295
            tunnel: w294 -> [w303 w326 w396 w405 w414 w422]
            tunnel: w289 -> [w301 w315 w401 w410 w419 w424]
            tunnel: [w300 w313 w399 w408 w417 w420] -> w284
            tunnel: w281 -> [_ w310 w398 w407 w416 _]
            frame "Idle", Default {
            }
            frame "generateWaves" {
              w319 = "Calculating" ("date/time string")
              n52 = Unbundle By Name(w312) -> ("Mode"=w325:T20)
              n53 = property on="Duration" class="Str"("Value"=w319) -> ()  [unwired: 2 in, 2 out]
              n54 = local write "Duration"(w319) -> ()
              n55 = case shown="\"Tweezers\"" w325 {
                tunnel: [w332 w342 w345 w353 w364 w369 w374] -> w308
                tunnel: w312 -> [_ w343 w346 w351 w360 w368 w383]
                tunnel: [w331 w341 w344 w352 w363 w370 w377] -> w309
                tunnel: w326 -> [w331 _ _ _ _ _ _]
                tunnel: w324 -> [w332 _ _ _ _ _ _]
                tunnel: w317 -> [w330 w340 w348 w350 w362 w372 w386]
                tunnel: w315 -> [w329 w339 w347 w349 w361 w371 w385]
                tunnel: [w328 w340 w348 w350 w362 w372 w386] -> w316
                tunnel: [w327 w339 w347 w349 w361 w371 w385] -> w314
                frame "X" {
                  n56 = disable-structure shown="Enabled" {
                    disable-tunnel: w330 -> [w336 w337]
                    disable-tunnel: w329 -> [w335 w338]
                    disable-tunnel: [w334 w338] -> w328
                    disable-tunnel: [w333 w337] -> w327
                    frame Enabled {
                      n57 = call "Calibration.vi"("Analogue In"=w336, "Digital In"=w335) -> ("Analogue In Out"=w333:refnum<k21>, "Digital Out"=w334:refnum<k21>)
                    }
                    frame Disabled {
                    }
                  }
                }
                frame "XY", Default {
                  n58 = call "XYWaveforms.vi"("Microscope Settings"=w343) -> ("Analogue Out"=w342:waveform(dbl)[], "Digital Out"=w341:digitalwaveform[])  [unwired: 1 out]
                }
                frame "XYZ" {
                  n59 = call "XYZWaveforms.vi"("Microscope Settings"=w346) -> ("Analogue Out out"=w345:waveform(dbl)[], "Digital Out out"=w344:digitalwaveform[])  [unwired: 2 in]
                }
                frame "XYZT" {
                  # "Creates delays by concatenating waveforms\nThis solution is slow and is more dangerous so probably shouldn't be used"
                  n60 = disable-structure shown="Enabled" {
                    disable-tunnel: [w356 w357] -> w353
                    disable-tunnel: [w355 w358] -> w352
                    disable-tunnel: w351 -> [w354 w359]
                    frame Disabled {
                      n61 = call "XYZTWaveforms.vi"("Microscope Settings"=w354) -> ("Digital Out"=w355:digitalwaveform[], "Analogue Out"=w356:waveform(dbl)[])  [unwired: 1 in]
                    }
                    frame Enabled {
                      n62 = call "XYZWaveforms.vi"("Microscope Settings"=w359) -> ("Analogue Out out"=w357:waveform(dbl)[], "Digital Out out"=w358:digitalwaveform[])  [unwired: 2 in]
                    }
                  }
                }
                frame "XYZC" {
                  n63 = call "XYZCWaveforms.vi"("Microscope Settings"=w360) -> ("Array"=w363:digitalwaveform[], "Analogue Out out"=w364:waveform(dbl)[])  [unwired: 1 in]
                }
                frame "Virus" {
                  n64 = Unbundle By Name(w368) -> ("ROI.Z"=w366:T1)
                  n65 = call "ImagetoZ.vi"("Z"=w366) -> ("ROI.Z"=w365:T1)  [unwired: 10 in]
                  n66 = Bundle By Name(cluster=w368, "ROI.Z"=w365) -> (w367:T2)
                  n67 = call "XYZWaveforms.vi"("Microscope Settings"=w367) -> ("Analogue Out out"=w369:waveform(dbl)[], "Digital Out out"=w370:digitalwaveform[])  [unwired: 2 in]
                }
                frame "Tweezers" {
                  n68 = Bundle By Name(cluster=w383, "Colour"=T15 [{"Laser"=enum."561", "Filter"=4}]) -> (w381:T2)
                  n69 = Bundle By Name(cluster=w381, "Colour"=T15 [{"Laser"=enum."488", "Filter"=4}], "ROI.Z"="Tweezers") -> (w380:T2)
                  n70 = call "XYZWaveforms.vi"("Microscope Settings"=w381) -> ("Analogue Out out"=w376:waveform(dbl)[], "Digital Out out"=w379:digitalwaveform[])  [unwired: 2 in]
                  n71 = call "XYZWaveforms.vi"("Microscope Settings"=w380) -> ("Analogue Out out"=w375:waveform(dbl)[], "Digital Out out"=w378:digitalwaveform[])  [unwired: 2 in]
                  n72 = for {
                    tunnel: w378 -> [w391] mode=indexing
                    tunnel: w379 -> [w392] mode=indexing
                    tunnel: [w390] -> w377 mode=indexing
                    n73 = call-poly <vilib>:"Append Digital Samples.vi"("digital waveform B"=w391, "digital waveform A"=w392) -> ("digital waveform out"=w390:digitalwaveform)  [unwired: 8 in, 1 out]
                  }
                  n74 = for {
                    tunnel: w375 -> [w388] mode=indexing
                    tunnel: w376 -> [w389] mode=indexing
                    tunnel: [w387] -> w374 mode=indexing
                    n75 = call-poly <vilib>:"Append Waveforms.vi"("waveform B"=w388, "waveform A"=w389) -> ("waveform out"=w387:waveform(dbl))  [unwired: 8 in, 1 out]
                  }
                }
              }
              n76 = Bundle By Name(cluster=w312, "Calibration Coordinates.Waveforms.Analogue Out"=w308, "Calibration Coordinates.Waveforms.Digital Out"=w309) -> (w311:T2)
              n77 = Bundle(Hardware."Update", "Microscope Settings"=w311) -> (w307:cluster{T8, "Microscope Settings":T2})  [unwired: 1 in]
              n78 = Enqueue Element(queue=w310, element=w307) -> ()  [unwired: 2 in, 3 out]
              n79 = Bundle("Analogue Out out"=w308, "Digital Out out"=w309) -> (w305:T22)  [unwired: 1 in]
              n80 = Index Array(array=w308) -> (element=w323:waveform(dbl))  [unwired: 1 in]
              n81 = call-poly <vilib>:"Waveform Duration.vi"("waveform in"=w323) -> ("duration"=w321:dbl)  [unwired: 8 in, 2 out]
              n82 = call "Graph.vi"("Cluster"=w305) -> ()
              n83 = To Time Stamp(1:w321) -> (0:w322:timestamp)
              n84 = Format Date/Time String(time format string (%c)="%H:%M:%S%4u", seconds (now)=w322) -> (date/time string=w318:string)  [unwired: 1 in]
              "Duration" <- w318
              n85 = property on="Duration" class="Str"("Value"=w318) -> ()  [unwired: 2 in, 2 out]
            }
            frame "runWaves" {
              n86 = Bundle(Hardware."Run Waves", "Microscope Settings"=w395) -> (w394:cluster{T8, "Microscope Settings":T2})  [unwired: 1 in]
              n87 = Enqueue Element(queue=w398, element=w394) -> ()  [unwired: 2 in, 3 out]
            }
            frame "runWavesCont" {
              n88 = Bundle(Hardware."RunCont", "Microscope Settings"=w404) -> (w403:cluster{T8, "Microscope Settings":T2})  [unwired: 1 in]
              n89 = Enqueue Element(queue=w407, element=w403) -> ()  [unwired: 2 in, 3 out]
            }
            frame "endWavesCont" {
              n90 = Bundle(Hardware."EndCont", "Microscope Settings"=w413) -> (w412:cluster{T8, "Microscope Settings":T2})  [unwired: 1 in]
              n91 = Enqueue Element(queue=w416, element=w412) -> ()  [unwired: 2 in, 3 out]
            }
            frame "stop" {
            }
          }
          n92 = local read "stop"() -> (w286:bool)
          n93 = Or(x=w287, y=w286) -> (x .or. y?=w285:bool)
          "Numeric 3" <- w280
        }
        n94 = call "IMAQ Create"("Image Name"="Images", "Image Type"=w166) -> ("New Image"=w176:T5, "error out"=w174:errorcluster)  [unwired: 3 in]
        n95 = while {
          tunnel: w186 -> [w746]
          shift-right: [w745] -> _
          shift-left: _ -> [w744]
          tunnel: w173 -> [w742]
          shift-right: [w741] -> _
          shift-left: w181 -> [w740]
          shift-right: [w739] -> w180
          shift-left: w179 -> [w738]
          stop <- w747 stop-if-true
          n96 = event shown="[16] \"Load Settings\": Value Change" {
            selector: _ -> [_ _ _ _ _ _ _ _ _ _ _ _ _ _ _ _ _]
            dyn-events: _ -> [_ _ _ _ _ _ _ _ _ _ _ _ _ _ _ _ _]
            timeout: 1 -> [_ _ _ _ _ _ _ _ _ _ _ _ _ _ _ _ _]
            tunnel: [w760 _ _ _ _ _ _ _ _ _ _ _ _ _ _ _ _] -> w747
            tunnel: w746 -> [w755 _ w779 w785 w796 _ w810 _ _ _ w846 _ _ _ _ _ _]
            tunnel: [w753 _ w773 w784 _ _ _ _ _ _ _ _ _ _ w900 _ w923] -> w745
            tunnel: w744 -> [w753 w767 w773 w784 w792 w801 w809 w823 w830 w836 w847 _ w867 w885 _ w904 w924]
            tunnel: w742 -> [w754 _ w778 _ w793 w802 _ w822 w826 w837 w845 _ w866 w884 _ _ _]
            tunnel: [w752 w762 w772 w782 w795 w805 w811 w821 w832 w839 w844 w855 w864 w882 w899 w905 w925] -> w741
            tunnel: w740 -> [w752 w764 w772 w782 w795 w805 w811 w821 w832 w839 w844 w855 w864 w882 w899 w905 w925]
            tunnel: [w748 w761 w768 w780 w787 w799 w807 w819 w828 w834 w840 w853 w863 w881 w898 w903 _] -> w739
            tunnel: w738 -> [w751 w761 w771 w781 w790 w800 w808 w820 w829 w833 w843 w852 w862 w880 w898 w901 _]
            event "stop": Value Change {
              w758 = ModeEnum."stop"  # Mode
              n97 = event-data() -> ()  [unwired: 1 in, 6 out]
              n98 = Bundle("Enum"=CameraControlTypeDef."Idle", "Value"=w753) -> (w756:cluster{"Enum":T14, "Value":T2})  [unwired: 1 in]
              n99 = Bundle("Mode"=w758, "Value"=w753) -> (w757:cluster{"Mode":T10, "Value":T2})  [unwired: 1 in]
              n100 = Enqueue Element(queue=w755, element=w756, error in (no error)=w751) -> (error out=w749:errorcluster)  [unwired: 1 in, 2 out]
              n101 = Enqueue Element(queue=w754, element=w757, error in (no error)=w751) -> (error out=w750:errorcluster)  [unwired: 1 in, 2 out]
              n102 = Merge Errors(w749, w750) -> (w748:errorcluster)
              n103 = local read "stop"() -> (w760:bool)
            }
            event Value Change {
              n104 = event-data() -> ()  [unwired: 1 in, 6 out]
              n105 = Flatten To XML(anything=w767) -> (xml string=w766:string)
              n106 = Build Array("Experiment 1" ("element"), w766) -> (w763:string[])
              n107 = Build Array (concatenate)(w764, w763) -> (w762:string[][])
              n108 = property on="Multicolumn Listbox" class="MCListbox (strict)"("ItemNames"=w762) -> ()  [unwired: 2 in, 2 out]
            }
            event Value Change {
              w776 = ModeEnum."generateWaves"  # Mode
              # "Live video for Calibration and 2D\nScan Modes.\n\nIdle Video for MultiD Scan modes\nUNTIL Begin Scan Button pressed?\n\nMultiD is waiting for trigger"
              n109 = event-data() -> ()  [unwired: 1 in, 6 out]
              n110 = Bundle("Enum"=CameraControlTypeDef."Trigger Source", "Value"=w773) -> (w774:cluster{"Enum":T14, "Value":T2})  [unwired: 1 in]
              n111 = Bundle("Mode"=w776, "Value"=w773) -> (w775:cluster{"Mode":T10, "Value":T2})  [unwired: 1 in]
              n112 = Enqueue Element(queue=w779, element=w774, error in (no error)=w771) -> (error out=w769:errorcluster)  [unwired: 1 in, 2 out]
              n113 = Enqueue Element(queue=w778, element=w775, error in (no error)=w771) -> (error out=w770:errorcluster)  [unwired: 1 in, 2 out]
              n114 = Merge Errors(w769, w770) -> (w768:errorcluster)
            }
            event Value Change {
              n115 = event-data() -> ()  [unwired: 1 in, 6 out]
              n116 = Bundle("Enum"=CameraControlTypeDef."Readout Mode", "Value"=w784) -> (w783:cluster{"Enum":T14, "Value":T2})  [unwired: 1 in]
              n117 = Enqueue Element(queue=w785, element=w783, error in (no error)=w781) -> (error out=w780:errorcluster)  [unwired: 1 in, 2 out]
            }
            event Value Change {
              w791 = ModeEnum."generateWaves"  # Mode
              n118 = event-data() -> ()  [unwired: 1 in, 6 out]
              n119 = Bundle("Enum"=CameraControlTypeDef."ROI", "Value"=w792) -> (w797:cluster{"Enum":T14, "Value":T2})  [unwired: 1 in]
              n120 = Bundle("Mode"=w791, "Value"=w792) -> (w794:cluster{"Mode":T10, "Value":T2})  [unwired: 1 in]
              n121 = Enqueue Element(queue=w796, element=w797, error in (no error)=w790) -> (error out=w788:errorcluster)  [unwired: 1 in, 2 out]
              n122 = Enqueue Element(queue=w793, element=w794, error in (no error)=w790) -> (error out=w789:errorcluster)  [unwired: 1 in, 2 out]
              n123 = Merge Errors(w788, w789) -> (w787:errorcluster)
            }
            event Value Change {
              w803 = ModeEnum."generateWaves"  # Mode
              n124 = event-data() -> ()  [unwired: 1 in, 6 out]
              n125 = Bundle("Mode"=w803, "Value"=w801) -> (w804:cluster{"Mode":T10, "Value":T2})  [unwired: 1 in]
              n126 = Enqueue Element(queue=w802, element=w804, error in (no error)=w800) -> (error out=w799:errorcluster)  [unwired: 1 in, 2 out]
            }
            event "Record": Value Change {
              n127 = event-data() -> ()  [unwired: 1 in, 6 out]
              n128 = case shown="True" "Record" {
                tunnel: w810 -> [_ w818]
                tunnel: w809 -> [_ w816]
                tunnel: w808 -> [w812 w814]
                tunnel: [w812 w813] -> w807
                frame False {
                }
                frame True {
                  n129 = Bundle("Enum"=CameraControlTypeDef."Ram Record", "Value"=w816) -> (w815:cluster{"Enum":T14, "Value":T2})  [unwired: 1 in]
                  n130 = Enqueue Element(queue=w818, element=w815, error in (no error)=w814) -> (error out=w813:errorcluster)  [unwired: 1 in, 2 out]
                }
              }
            }
            event Value Change {
              w825 = ModeEnum."generateWaves"  # Mode
              n131 = event-data() -> ()  [unwired: 1 in, 6 out]
              n132 = Bundle("Mode"=w825, "Value"=w823) -> (w824:cluster{"Mode":T10, "Value":T2})  [unwired: 1 in]
              n133 = Enqueue Element(queue=w822, element=w824, error in (no error)=w820) -> (error out=w819:errorcluster)  [unwired: 1 in, 2 out]
            }
            event Value Change {
              w831 = ModeEnum."generateWaves"  # Mode
              n134 = event-data() -> ()  [unwired: 1 in, 6 out]
              n135 = Bundle("Mode"=w831, "Value"=w830) -> (w827:cluster{"Mode":T10, "Value":T2})  [unwired: 1 in]
              n136 = Enqueue Element(queue=w826, element=w827, error in (no error)=w829) -> (error out=w828:errorcluster)  [unwired: 1 in, 2 out]
            }
            event Value Change {
              w838 = ModeEnum."generateWaves"  # Mode
              n137 = event-data() -> ()  [unwired: 1 in, 6 out]
              n138 = Bundle("Mode"=w838, "Value"=w836) -> (w835:cluster{"Mode":T10, "Value":T2})  [unwired: 1 in]
              n139 = Enqueue Element(queue=w837, element=w835, error in (no error)=w833) -> (error out=w834:errorcluster)  [unwired: 1 in, 2 out]
            }
            event Value Change {
              w850 = ModeEnum."generateWaves"  # Mode
              n140 = event-data() -> ()  [unwired: 1 in, 6 out]
              n141 = Bundle("Enum"=CameraControlTypeDef."Update", "Value"=w847) -> (w848:cluster{"Enum":T14, "Value":T2})  [unwired: 1 in]
              n142 = Bundle("Mode"=w850, "Value"=w847) -> (w849:cluster{"Mode":T10, "Value":T2})  [unwired: 1 in]
              n143 = Enqueue Element(queue=w846, element=w848, error in (no error)=w843) -> (error out=w842:errorcluster)  [unwired: 1 in, 2 out]
              n144 = Enqueue Element(queue=w845, element=w849, error in (no error)=w843) -> (error out=w841:errorcluster)  [unwired: 1 in, 2 out]
              n145 = Merge Errors(w842, w841) -> (w840:errorcluster)
            }
            event "Signals Debugger": Value Change {
              n146 = event-data() -> ()  [unwired: 1 in, 6 out]
              n147 = case shown="True" "Signals Debugger" {
                tunnel: [w856 w858] -> w853
                tunnel: w852 -> [w856 w857]
                frame False {
                }
                frame True {
                  n148 = vi-ref "Graph.vi"() -> (w859:refnum<vi>)
                  n149 = invoke class="VI" method="FP.Open"(reference=w859, error in=w857, "Activate"=TRUE ("Front Panel Window:Open"), "State"=T16."Standard") -> (error out=w858:errorcluster)  [unwired: 1 in, 4 out]
                }
              }
            }
            event "Scan": Value Change {
              n150 = event-data() -> ("NewVal"=w865:bool)  [unwired: 1 in, 5 out]
              n151 = case shown="True" w865 {
                tunnel: w867 -> [_ w873]
                tunnel: w866 -> [_ w872]
                tunnel: [w868 w871] -> w863
                tunnel: w862 -> [w868 w870]
                frame False {
                }
                frame True {
                  n152 = for {
                    N: "Scans" -> [_]
                    tunnel: w873 -> [w876]
                    tunnel: w872 -> [w879]
                    tunnel: [w875] -> w871
                    tunnel: w870 -> [w874]
                    w878 = ModeEnum."runWaves"  # Mode
                    n153 = Bundle("Mode"=w878, "Value"=w876) -> (w877:cluster{"Mode":T10, "Value":T2})  [unwired: 1 in]
                    n154 = Enqueue Element(queue=w879, element=w877, error in (no error)=w874) -> (error out=w875:errorcluster)  [unwired: 1 in, 2 out]
                  }
                }
              }
            }
            event "Scan Cont": Value Change {
              n155 = event-data() -> ("NewVal"=w883:bool)  [unwired: 1 in, 5 out]
              n156 = case shown="True" w883 {
                tunnel: w885 -> [w891 w897]
                tunnel: w884 -> [w890 w896]
                tunnel: [w889 w895] -> w881
                tunnel: w880 -> [w888 w894]
                frame True {
                  w887 = ModeEnum."runWavesCont"  # Mode
                  n157 = Bundle("Mode"=w887, "Value"=w891) -> (w886:cluster{"Mode":T10, "Value":T2})  [unwired: 1 in]
                  n158 = Enqueue Element(queue=w890, element=w886, error in (no error)=w888) -> (error out=w889:errorcluster)  [unwired: 1 in, 2 out]
                }
                frame False {
                  w893 = ModeEnum."endWavesCont"  # Mode
                  n159 = Bundle("Mode"=w893, "Value"=w897) -> (w892:cluster{"Mode":T10, "Value":T2})  [unwired: 1 in]
                  n160 = Enqueue Element(queue=w896, element=w892, error in (no error)=w894) -> (error out=w895:errorcluster)  [unwired: 1 in, 2 out]
                }
              }
            }
            event Timeout {
              n161 = event-data() -> ()  [unwired: 1 in, 3 out]
              n162 = property on="Microscope Settings" class="Clust (strict)"() -> ("Value"=w900:T2)  [unwired: 2 in, 2 out]
            }
            event "Save Settings": Value Change {
              n163 = event-data() -> ("NewVal"=w902:bool)  [unwired: 1 in, 5 out]
              n164 = case shown="True" w902 {
                tunnel: w904 -> [_ w921]
                tunnel: [w906 w909] -> w903
                tunnel: w901 -> [w906 _]
                frame False {
                }
                frame True {
                  n165 = Flatten To XML(anything=w921) -> (xml string=w914:string)
                  n166 = call "File Dialog"("start path"=path "C:/_DATA", "prompt"="Save your Settings", "button label"="Save", "default name"="SpimSettings", "pattern (all files)"=".xml") -> ("selected path"=w915:path, "error out"=w908:errorcluster)  [unwired: 7 in, 2 out]
                  n167 = Open/Create/Replace File(file path (use dialog)=w915, error in=w908, operation (0:open)=T17."replace or create with confirmation") -> (refnum out=w913:refnum<file>, error out=w910:errorcluster)  [unwired: 3 in, 1 out]
                  n168 = Write to Text File(file (use dialog)=w913, text=w914, error in=w910) -> (refnum out=w912:refnum<file>, error out=w911:errorcluster)  [unwired: 1 in, 1 out]
                  n169 = Close File(refnum=w912, error in=w911) -> (error out=w909:errorcluster)  [unwired: 1 out]
                }
              }
            }
            event "Load Settings": Value Change {
              n170 = event-data() -> ("NewVal"=w922:bool)  [unwired: 1 in, 5 out]
              n171 = case shown="True" w922 {
                tunnel: w924 -> [w926 w929]
                tunnel: [w926 w928] -> w923
                frame False {
                }
                frame True {
                  (unwired) "Load your Settings" ("prompt")
                  n172 = call "File Open"("start path"=path "C:/_DATA", "button label"="Load", "default name"="SpimSettings", "pattern (all files)"="*.xml") -> ("selected path"=w930:path, "cancelled"=w927:bool)  [unwired: 8 in, 2 out]
                  n173 = case shown="False" w927 {
                    tunnel: w930 -> [_ w940]
                    tunnel: w929 -> [w935 w938]
                    tunnel: [w935 w936] -> w928
                    frame True {
                    }
                    frame False {
                      n174 = Read from Text File(file (use dialog)=w940) -> (text=w939:string, error out=w937:errorcluster)  [unwired: 3 in, 2 out]
                      n175 = Unflatten From XML(xml string=w939, type=w938, error in (no error)=w937) -> (value=w936:T2)  [unwired: 1 out]
                      n176 = property on="Microscope Settings" class="Clust (strict)"("Val(Sgnl)"=w936) -> ()  [unwired: 2 in, 2 out]
                    }
                  }
                }
              }
            }
          }
        }
        n177 = while "Camera Consumer" {
          tunnel: w179 -> [w505]
          tunnel: [w509] -> w195
          tunnel: w186 -> [w516]
          tunnel: [w523] -> w194
          shift-right: [w522] -> _
          shift-left: CameraControlTypeDef."Preview" ("Enum") -> [w513]
          tunnel: [w519] -> w190
          tunnel: w189 -> [w518]
          tunnel: w187 -> [w512]
          shift-right: [w520] -> w198
          shift-left: w199 -> [w521]
          tunnel: w173 -> [w507]
          stop <- w508 stop-if-true
          n178 = Dequeue Element(queue=w516, timeout in ms (-1)=1, error in (no error)=w505) -> (queue out=w515:refnum<queue>, element=w511:cluster{"Enum":T14, "Microscope Settings":T2}, timed out?=w504:bool, error out=w506:errorcluster)
          n179 = case shown="False" w504 {
            tunnel: [w525 CameraControlTypeDef."Preview" ("Enum")] -> w514
            tunnel: w513 -> [_ _]
            tunnel: w511 -> [w526 _]
            tunnel: [w524 _] -> w510
            frame False {
              n180 = Unbundle(w526) -> ("Enum"=w525:T14, "Microscope Settings"=w524:T2)
            }
            frame True {
            }
          }
          n181 = case shown="\"Ram Record\"" w514 {
            selector: w514 -> [w531 w536 w568 w591 w596 w607 w612 w617 w622 w627 w660 w678 _ w706 _]
            tunnel: w515 -> [w530 w537 w569 w592 w597 w608 w613 w618 w623 w628 _ w674 w688 w708 w727]
            tunnel: [w530 w537 w569 w592 w597 w608 w613 w618 w623 w628 _ w674 w688 w708 w727] -> w523
            tunnel: w506 -> [w532 w535 w567 w590 w595 w606 w611 w616 w621 w626 w655 w677 w681 w705 w718]
            tunnel: [w532 w535 w544 w590 w595 w606 w611 w616 w621 w626 w629 w677 w680 w705 w719] -> w509
            tunnel: [w531 w536 w568 w591 w596 w607 w612 w617 w622 w627 w660 w678 CameraControlTypeDef."Preview" ("Enum") w706 w709] -> w522
            tunnel: w521 -> [w529 w534 w551 w589 w593 w604 w610 w615 w620 w625 w657 w676 w687 w707 w721]
            tunnel: [w529 w534 w550 w589 w593 w603 w610 w615 w620 w625 w631 w676 w685 w707 w720] -> w520
            tunnel: [w528 w533 w546 w588 w594 w605 w609 w614 w619 w624 w659 w675 w683 w704 w722] -> w519
            tunnel: w518 -> [w528 w533 _ w588 w594 w605 w609 w614 w619 w624 w659 w675 w683 w704 _]
            tunnel: w512 -> [_ _ w560 _ _ _ _ _ _ _ _ _ w682 _ _]
            tunnel: w510 -> [_ _ w539 _ _ w602 _ _ _ _ w654 _ _ _ w711]
            tunnel: w507 -> [_ _ w540 _ _ _ _ _ _ _ _ _ _ _ _]
            frame "Idle" {
            }
            frame "IntervalLineInt" {
            }
            frame "Ram Record" {
              w564 = 0 items=["Snap", "Sequence"] ("Capture mode")
              w547 = 1 items=["Snap", "Sequence"] ("Capture mode")
              n182 = call "tm_stopcapture.vi"("error in (no error)"=w567, "Handle in"=w551) -> ("error out"=w542:errorcluster, "Handle out"=w543:u32)  [unwired: 8 in]
              n183 = call "tm_unpreparecapture.vi"("error in (no error)"=w542, "Handle in"=w543) -> ("error out"=w566:errorcluster, "Handle out"=w565:u32)  [unwired: 8 in]
              n184 = call "tm_preparecapture.vi"("error in (no error)"=w566, "Frames"="Frames", "Capture mode"=w564, "Handle in"=w565) -> ("error out"=w562:errorcluster, "Buffer Info"=w548:T7, "Handle out"=w563:u32)  [unwired: 4 in, 1 out]
              n185 = call "tm_startcapture_b.vi"("error in (no error)"=w562, "Handle in"=w563) -> ("error out"=w541:errorcluster, "Handle out"=w561:u32)  [unwired: 8 in]
              n186 = for {
                N: "Frames" -> [_]
                tunnel: w541 -> [w587]
                tunnel: w561 -> [w586]
                tunnel: w560 -> [w582]
                tunnel: [w580] -> w556
                tunnel: [w579] -> w555
                tunnel: w548 -> [w578]
                tunnel: w541 -> [w575]
                tunnel: w540 -> [w574]
                tunnel: w539 -> [_]
                tunnel: w539 -> [w572]
                tunnel: [w571] -> w538 mode=indexing
                n187 = call "tm_waitnextframe.vi"("error in (no error)"=w587, "Handle in"=w586) -> ("error out"=w585:errorcluster, "Handle out"=w584:u32)  [unwired: 6 in, 2 out]
                n188 = call "tm_getframe_a.vi"("error in (no error)"=w585, "Buffer Info"=w578, "Handle in"=w584) -> ("error out"=w580:errorcluster, "Data 16"=w576:u16[][], "Handle out"=w579:u32)  [unwired: 4 in, 2 out]
                n189 = Bundle("Mode"=ModeEnum."runWaves", "Microscope Settings"=w572) -> (w570:cluster{"Mode":T10, "Microscope Settings":T2})  [unwired: 1 in]
                n190 = Enqueue Element(queue=w574, element=w570, error in (no error)=w575) -> (error out=w571:errorcluster)  [unwired: 1 in, 2 out]
                n191 = Bundle By Name(cluster=T12 {"State"=enum."Start Sequence", "Stack Number"=0, "Image"=[], "Stacks"=0} ("element"), "State"=Stack_Track."Save Image", "Image"=w576) -> (w581:T12)
                n192 = Enqueue Element(queue=w582, element=w581) -> ()  [unwired: 2 in, 3 out]
              }
              n193 = call "tm_stopcapture.vi"("error in (no error)"=w556, "Handle in"=w555) -> ("error out"=w557:errorcluster, "Handle out"=w554:u32)  [unwired: 8 in]
              n194 = call "tm_unpreparecapture.vi"("error in (no error)"=w557, "Handle in"=w554) -> ("error out"=w558:errorcluster, "Handle out"=w553:u32)  [unwired: 8 in]
              n195 = call "tm_preparecapture.vi"("error in (no error)"=w558, "Capture mode"=w547, "Handle in"=w553) -> ("error out"=w559:errorcluster, "Buffer Info"=w546:T7, "Handle out"=w552:u32)  [unwired: 5 in, 1 out]
              n196 = call "tm_startcapture_b.vi"("error in (no error)"=w559, "Handle in"=w552) -> ("error out"=w545:errorcluster, "Handle out"=w550:u32)  [unwired: 8 in]
              n197 = Merge Errors(w538, w545) -> (w544:errorcluster)
            }
            frame "HardDisk Record" {
            }
            frame "Disengage Update" {
            }
            frame "Update", Default {
              w599 = u32 2049184 items=["SENSOR MODE"=4212128, "CCD MODE"=4212384, "READOUT MODE"=4211872, "ACTIVE VIEW INDEX"=4343136, "BITS PER CHANNEL"=4342976, "IMAGE PIXEL TYPE"=4343296, "BINNING"=4215968, "EXPOSURE TIME"=2049184, "CONTRAST GAIN"=3163312, "CONTRAST OFFSET"=3163328, "LIGHT MODE"=2114720, "SENSITIVITY"=2114992, "PHOTON IMAGING MODE"=2115200, "HIGH DYNAMIC RANGE MODE"=3163360, "WHITE BALANCE"=3163568, "TEMPERATURE"=2115232, "TEMPERATURE TARGET"=2115264, "SENSOR COOLER FAN"=2115296, "LINEBUNDLE HEIGHT"=4212192, "MECHANICAL SHUTTER"=2115488, "BACK FOCUS POSITION"=8422304, "TRIGGER CONNECTOR"=1066432, "TRIGGER SOURCE"=1066144, "OUTPUT TRIGGER SOURCE"=1852576, "TRIGGER GLOBAL EXPOSURE"=2049680, "FIRST TRIGGER BEHAVIOR"=2049696, "CHANNEL SYNC"=1852352, "READOUT DIRECTION"=4211904, "PRE HSYNC COUNT"=1852704, "INTERNAL LINE SPEED"=4226000, "INTERNAL LINE INTERVAL"=4226016] ("Parameter")
              n198 = Unbundle By Name(w602) -> ("Exposure/ms"=w601:dbl)  [unwired: 1 out]
              n199 = Divide(x=w601, y=1000.0) -> (x/y=w598:dbl)
              n200 = call "tm_setparameter_a.vi"("Value in"=w598, "Parameter"=w599, "Handle in"=w604) -> ("Handle out"=w603:u32)  [unwired: 7 in, 1 out]
            }
            frame "ROI" {
            }
            frame "Binning" {
            }
            frame "Scan Mode" {
            }
            frame "Trigger Mode" {
            }
            frame "Readout Mode" {
              w635 = 1 items=["Snap", "Sequence"] ("Capture mode")
              w641 = u32 4194832  # Sensor Mode
              w644 = u32 2031888  # Exposure time
              n201 = Unbundle By Name(w654) -> ("Exposure/ms"=w653:dbl, "Slit.Slit Width /%"=w649:dbl, "Slit.Scanning Mode"=w639:dbl)
              n202 = call "tm_stopcapture.vi"("error in (no error)"=w655, "Handle in"=w657) -> ("error out"=w658:errorcluster, "Handle out"=w656:u32)  [unwired: 8 in]
              n203 = Divide(x=w653, y=1000.0) -> (x/y=w651:dbl)
              n204 = Multiply(x=w649, y=2048 ("input variable")) -> (x*y=w648:dbl)
              n205 = call "tm_unpreparecapture.vi"("error in (no error)"=w658, "Handle in"=w656) -> ("error out"=w636:errorcluster, "Handle out"=w640:u32)  [unwired: 8 in]
              n206 = call "tm_setpropertyvalue.vi"("error in (no error)"=w636, "Value in"=w639, "Property ID"=w641, "Handle in"=w640) -> ("error out"=w637:errorcluster, "Handle out"=w638:u32)  [unwired: 6 in]
              n207 = Divide(x=w648, y=100.0) -> (x/y=w646:dbl)
              n208 = case shown="1, Default" w639 {
                tunnel: [w663 w664] -> w645
                tunnel: w651 -> [w663 w672]
                tunnel: w646 -> [_ w671]
                tunnel: w638 -> [w662 w666]
                tunnel: [w662 w668] -> w643
                tunnel: [w661 w667] -> w642
                tunnel: w637 -> [w661 w665]
                frame 1, Default {
                }
                frame 12 {
                  w670 = u32 4208720  # Line Interval
                  n209 = formula code="slitExpos=frameInter*LW/(LinesToReadout\n+10+LW);\nlineInter = slitExpos / LW;"("frameInter"=w672, "LW"=w671, "LinesToReadout"=2048 ("input variable")) -> ("slitExpos"=w664:dbl, "lineInter"=w669:dbl)
                  n210 = call "tm_setpropertyvalue.vi"("error in (no error)"=w665, "Value in"=w669, "Property ID"=w670, "Handle in"=w666) -> ("error out"=w667:errorcluster, "Handle out"=w668:u32)  [unwired: 6 in]
                }
              }
              n211 = call "tm_setpropertyvalue.vi"("error in (no error)"=w642, "Value in"=w645, "Property ID"=w644, "Handle in"=w643) -> ("error out"=w630:errorcluster, "Handle out"=w632:u32)  [unwired: 6 in]
              n212 = call "tm_preparecapture.vi"("error in (no error)"=w630, "Capture mode"=w635, "Handle in"=w632) -> ("error out"=w634:errorcluster, "Handle out"=w633:u32)  [unwired: 5 in, 2 out]
              n213 = call "tm_startcapture_b.vi"("error in (no error)"=w634, "Handle in"=w633) -> ("error out"=w629:errorcluster, "Handle out"=w631:u32)  [unwired: 8 in]
            }
            frame "Readout Direction" {
            }
            frame "Preview" {
              (unwired) 500 ("Timeout")
              n214 = call "tm_waitnextframe.vi"("error in (no error)"=w681, "Handle in"=w687) -> ("error out"=w679:errorcluster, "Handle out"=w686:u32)  [unwired: 6 in, 2 out]
              n215 = case shown="No Error" w679 {
                selector: w679 -> [w689 w703]
                tunnel: w686 -> [w701 w702]
                tunnel: [w700 w702] -> w685
                tunnel: w683 -> [w699 _]
                tunnel: w682 -> [w698 _]
                tunnel: w681 -> [w693 _]
                tunnel: [w690 w703] -> w680
                frame No Error {
                  w695 = 0 ("Timeout")
                  n216 = call "tm_getframe_a.vi"("error in (no error)"=w689, "Buffer Info"=w699, "Handle in"=w701) -> ("error out"=w691:errorcluster, "Data 16"=w696:u16[][], "Handle out"=w700:u32)  [unwired: 4 in, 2 out]
                  n217 = Bundle("State"=Stack_Track."Display", "Timeout"=w695, "Data 16"=w696, "Timeout"=w695) -> (w694:T23)  [unwired: 1 in]
                  n218 = Enqueue Element(queue=w698, element=w694, error in (no error)=w693) -> (error out=w692:errorcluster)  [unwired: 1 in, 2 out]
                  n219 = Merge Errors(w691, w692) -> (w690:errorcluster)
                }
                frame Error {
                }
              }
            }
            frame "ROIWindow" {
            }
            frame "Trigger Source" {
              (unwired) u32 1066144 items=["SENSOR MODE"=4212128, "CCD MODE"=4212384, "READOUT MODE"=4211872, "ACTIVE VIEW INDEX"=4343136, "BITS PER CHANNEL"=4342976, "IMAGE PIXEL TYPE"=4343296, "BINNING"=4215968, "EXPOSURE TIME"=2049184, "CONTRAST GAIN"=3163312, "CONTRAST OFFSET"=3163328, "LIGHT MODE"=2114720, "SENSITIVITY"=2114992, "PHOTON IMAGING MODE"=2115200, "HIGH DYNAMIC RANGE MODE"=3163360, "WHITE BALANCE"=3163568, "TEMPERATURE"=2115232, "TEMPERATURE TARGET"=2115264, "SENSOR COOLER FAN"=2115296, "LINEBUNDLE HEIGHT"=4212192, "MECHANICAL SHUTTER"=2115488, "BACK FOCUS POSITION"=8422304, "TRIGGER CONNECTOR"=1066432, "TRIGGER SOURCE"=1066144, "OUTPUT TRIGGER SOURCE"=1852576, "TRIGGER GLOBAL EXPOSURE"=2049680, "FIRST TRIGGER BEHAVIOR"=2049696, "CHANNEL SYNC"=1852352, "READOUT DIRECTION"=4211904, "PRE HSYNC COUNT"=1852704, "INTERNAL LINE SPEED"=4226000, "INTERNAL LINE INTERVAL"=4226016] ("Parameter")
              w717 = 1 items=["Snap", "Sequence"] ("Capture mode")
              n220 = Unbundle By Name(w711) -> ("Mode"=w710:T20)
              n221 = call "tm_stopcapture.vi"("error in (no error)"=w718, "Handle in"=w721) -> ("error out"=w725:errorcluster, "Handle out"=w726:u32)  [unwired: 8 in]
              n222 = call "tm_unpreparecapture.vi"("error in (no error)"=w725, "Handle in"=w726) -> ("error out"=w713:errorcluster, "Handle out"=w716:u32)  [unwired: 8 in]
              n223 = case shown="\"XY\", Default" w710 {
                tunnel: [T11 {"Mode"=2, "Polarity"=2, "Times"=2, "Delay"=0.0} ("Parameters") T11 {"Mode"=2, "Polarity"=2, "Times"=2, "Delay"=0.0} ("Parameters") T11 {"Mode"=2, "Polarity"=2, "Times"=2, "Delay"=0.0} ("Parameters") T11 {"Mode"=1, "Polarity"=2, "Times"=2, "Delay"=0.0} ("Parameters") T11 {"Mode"=1, "Polarity"=2, "Times"=2, "Delay"=0.0} ("Parameters")] -> w714
                tunnel: [CameraControlTypeDef."Preview" ("Enum") CameraControlTypeDef."Idle" ("Enum") CameraControlTypeDef."Idle" ("Enum") CameraControlTypeDef."Idle" ("Enum") CameraControlTypeDef."Preview" ("Enum")] -> w709
                frame "XY", Default {
                }
                frame "XYZT" {
                }
                frame "XYZ" {
                }
                frame "XYZC" {
                }
                frame "X" {
                }
              }
              n224 = call "tm_setinputtrigger.vi"("error in (no error)"=w713, "Parameters"=w714, "Handle in"=w716) -> ("error out"=w712:errorcluster, "Handle out"=w715:u32)  [unwired: 7 in]
              n225 = call "tm_preparecapture.vi"("error in (no error)"=w712, "Capture mode"=w717, "Handle in"=w715) -> ("error out"=w724:errorcluster, "Buffer Info"=w722:T7, "Handle out"=w723:u32)  [unwired: 5 in, 1 out]
              n226 = call "tm_startcapture_b.vi"("error in (no error)"=w724, "Handle in"=w723) -> ("error out"=w719:errorcluster, "Handle out"=w720:u32)  [unwired: 8 in]
            }
          }
          n227 = local read "stop"() -> (w508:bool)
        }
        n228 = while "Tiff Consumer" {
          tunnel: [w442] -> w193
          tunnel: w187 -> [w443]
          shift-right: [w436] -> _
          shift-left: w176 -> [w433]
          shift-right: [w431] -> _
          shift-left: u32[] [] -> [w432]
          shift-right: [w434] -> w196
          shift-left: w174 -> [w430]
          shift-right: [w427] -> _
          shift-left: T12 {"State"=enum."Idle", "Stack Number"=0, "Image"=[], "Stacks"=0} ("input cluster") -> [w426]
          i -> [w429]
          stop <- w445 stop-if-true
          # "Delay, maybe?\nCheck"
          n229 = Unbundle By Name(w426) -> ("State"=w438:T13, "Stack Number"=→"Stack Number":i32, "Image"=w439:u16[][])
          n230 = Dequeue Element(queue=w443, timeout in ms (-1)=1, error in (no error)=w430) -> (queue out=w441:refnum<queue>, element=w427:T12, error out=w440:errorcluster)  [unwired: 1 out]
          n231 = case shown="\"STOP\"" w438 {
            tunnel: [w458 w474 w477 w482 w486 w490 w494 w503] -> w442
            tunnel: w441 -> [w458 w474 w477 w482 w486 w490 w494 w503]
            tunnel: w439 -> [w448 _ _ _ _ _ _ w502]
            tunnel: w433 -> [w446 w472 w476 w480 w484 w488 w492 w500]
            tunnel: w440 -> [w457 w473 w478 w481 w485 w489 w493 w501]
            tunnel: [w456 w473 w478 w481 w485 w489 w493 w496] -> w435
            tunnel: [w447 w472 w476 w480 w484 w488 w492 w497] -> w436
            tunnel: w432 -> [w455 w471 w475 w479 w483 w487 w491 w495]
            tunnel: [w450 w471 w475 w479 w483 w487 w491 w495] -> w431
            frame "Display" {
              w451 = 10 ("y")
              n232 = Add Array Elements(numeric array=w448) -> ()  [unwired: 1 out]
              n233 = call "IMAQ ArrayToImage"("Image Pixels (U16)"=w448, "error in (no error)"=w457, "Image"=w446) -> ("error out"=w456:errorcluster, "Image Out"=w447:T5)  [unwired: 7 in]
              n234 = Tick Count (ms)() -> (millisecond timer value=w449:u32)
              n235 = Build Array (concatenate)(w455, w449) -> (w452:u32[])
              n236 = Array Size(array=w452) -> (size(s)=w454:i32)
              n237 = Greater?(x=w454, y=w451) -> (0:w453:bool)
              n238 = case shown="True" w453 {
                tunnel: w452 -> [w459 w462]
                tunnel: w451 -> [_ w469]
                tunnel: [w459 w460] -> w450
                frame False {
                }
                frame True {
                  n239 = Array Subset(array=w462, index=1, length=w469) -> (w460:u32[])
                  n240 = Index Array(array=w460, index=0) -> (element=w466:u32)
                  n241 = Index Array(array=w460, index=9) -> (element=w467:u32)
                  n242 = Subtract(x=w467, y=w466) -> (x-y=w465:u32)
                  n243 = Divide(x=10000.0, y=w465) -> (x/y=→"FPS":dbl)
                }
              }
            }
            frame "Idle", Default {
            }
            frame "Start Sequence" {
            }
            frame "Read Disk" {
            }
            frame "STOP" {
            }
            frame "Collecting" {
            }
            frame "End" {
            }
            frame "Save Image" {
              n244 = call "4Digit File Incrementer.vi"("path"="Save to:") -> ("appended path"=w498:path)  [unwired: 10 in]
              n245 = call "IMAQ ArrayToImage"("Image Pixels (U16)"=w502, "error in (no error)"=w501, "Image"=w500) -> ("error out"=w496:errorcluster, "Image Out"=w497:T5)  [unwired: 7 in]
              n246 = local write "Save to:"(w498) -> ()
              n247 = call-poly "IMAQ Write File 2"("error in (no error)"=w496, "File Path"=w498, "Image"=w497) -> ()  [unwired: 7 in, 2 out]
            }
          }
          "Image" <- w436
          n248 = call "IMAQ Histograph"("error in (no error)"=w435, "Image"=w436) -> ("error out"=w434:errorcluster, "Histogram Graph"=→"Histogram":T6)  [unwired: 6 in, 2 out]
          n249 = local read "stop"() -> (w445:bool)
          "Numeric" <- w429
        }
        n250 = while {
          tunnel: [w223] -> w168
          tunnel: w167 -> [w222]
          shift-right: [w219] -> _
          shift-left: w170 -> [w217]
          shift-right: [w218] -> _
          shift-left: w169 -> [w216]
          shift-right: [w210] -> _
          shift-left: w171 -> [w212]
          shift-right: [w211] -> _
          shift-left: w172 -> [w213]
          shift-right: [w205] -> _
          shift-left: _ -> [w207]
          shift-right: [w202] -> _
          shift-left: _ -> [w200]
          i -> [w209]
          stop <- w215 stop-if-true
          n251 = Dequeue Element(queue=w222, timeout in ms (-1)=1) -> (queue out=w221:refnum<queue>, element=w220:cluster{T8, "Microscope Settings":T2}, timed out?=w206:bool)  [unwired: 1 in, 1 out]
          n252 = case shown="\"Update\"" w207 {
            tunnel: [w235 w243 w245 w257 w262 w275] -> w223
            tunnel: w221 -> [w235 w243 w245 w257 w262 w275]
            tunnel: w200 -> [_ w239 w249 _ w266 _]
            tunnel: [w234 w238 w250 w259 w267 w277] -> w219
            tunnel: [w233 w237 w251 w260 w268 w276] -> w218
            tunnel: w217 -> [w234 _ w250 w259 w267 w277]
            tunnel: w216 -> [w233 _ w251 w260 w268 w276]
            tunnel: [FALSE FALSE FALSE FALSE FALSE FALSE] -> w214
            tunnel: w213 -> [w232 w242 w253 w256 w270 w273]
            tunnel: w212 -> [w231 w241 w252 w255 w269 w272]
            tunnel: [w232 w242 w248 w256 w265 w273] -> w211
            tunnel: [w231 w241 w247 w255 w264 w272] -> w210
            tunnel: [Hardware."Idle" Hardware."Idle" Hardware."Idle" Hardware."Idle" Hardware."RunCont" Hardware."Idle"] -> w204
            frame "Idle", Default {
            }
            frame "Update" {
              n253 = Unbundle By Name(w239) -> ("Calibration Coordinates.Waveforms.Analogue Out"=w238:waveform(dbl)[], "Calibration Coordinates.Waveforms.Digital Out"=w237:digitalwaveform[])
              n254 = Bundle("Analogue Out"=w238, "Digital Out"=w237) -> ()  [unwired: 1 in, 1 out]
            }
            frame "Run Waves" {
              n255 = call "RunWaves.vi"("Analogue Out"=w250, "Digital Out"=w251, "Microscope Settings"=w249, "Mirror Z in"=w252, "Refnum in"=w253) -> ("task out"=w247:refnum<k21>, "Refnum out"=w248:refnum<k21>)  [unwired: 5 in]
            }
            frame "EndCont" {
            }
            frame "RunCont" {
              n256 = call "RunWaves.vi"("Analogue Out"=w267, "Digital Out"=w268, "Microscope Settings"=w266, "Mirror Z in"=w269, "Refnum in"=w270) -> ("task out"=w264:refnum<k21>, "Refnum out"=w265:refnum<k21>)  [unwired: 5 in]
            }
            frame "Stop" {
            }
          }
          n257 = Unbundle(w220) -> (w201:T8, "Microscope Settings"=w203:T2)
          n258 = case shown="True" w206 {
            tunnel: [w225 w228] -> w205
            tunnel: w204 -> [_ w228]
            tunnel: [w226 w227] -> w202
            tunnel: w203 -> [w226 _]
            tunnel: w201 -> [w225 _]
            tunnel: w200 -> [_ w227]
            frame False {
            }
            frame True {
            }
          }
          n259 = local read "stop"() -> (w224:bool)
          n260 = Or(x=w214, y=w224) -> (x .or. y?=w215:bool)
          "Numeric 2" <- w209
        }
        n261 = Merge Errors(w180, w195, w196) -> (w197:errorcluster)
      }
      frame "deinit" {
        n262 = call <vilib>:"DAQmx Stop Task.vi"("task/channels in"=w952) -> ("task out"=w953:refnum<k21>)  [unwired: 13 in, 1 out]
        n263 = call <vilib>:"DAQmx Stop Task.vi"("task/channels in"=w954) -> ("task out"=w955:refnum<k21>)  [unwired: 13 in, 1 out]
        n264 = call <vilib>:"DAQmx Clear Task.vi"("task in"=w953) -> ("error out"=w949:errorcluster)  [unwired: 14 in]
        n265 = call "tm_stopcapture.vi"("error in (no error)"=w963, "Handle in"=w959) -> ("error out"=w966:errorcluster, "Handle out"=w965:u32)  [unwired: 8 in]
        n266 = call <vilib>:"DAQmx Clear Task.vi"("task in"=w955) -> ("error out"=w950:errorcluster)  [unwired: 14 in]
        n267 = call "tm_unpreparecapture.vi"("error in (no error)"=w966, "Handle in"=w965) -> ("error out"=w967:errorcluster, "Handle out"=w964:u32)  [unwired: 8 in]
        n268 = call "tm_closecamera.vi"("error in (no error)"=w967, "Handle in"=w964) -> ("error out"=w968:errorcluster)  [unwired: 9 in]
        n269 = Flush Queue(queue=w942) -> (queue out=w948:refnum<queue>)  [unwired: 1 in, 2 out]
        n270 = call "tm_deinitialize.vi"("error in (no error)"=w968) -> ("error out"=w945:errorcluster)  [unwired: 10 in]
        n271 = Release Queue(queue=w943, error in (no error)=w945) -> (error out=w961:errorcluster)  [unwired: 1 in, 2 out]
        n272 = Release Queue(queue=w948) -> (error out=w951:errorcluster)  [unwired: 2 in, 2 out]
        n273 = Flush Queue(queue=w947, error in (no error)=w945) -> (queue out=w946:refnum<queue>, error out=w944:errorcluster)  [unwired: 1 out]
        n274 = Release Queue(queue=w946, error in (no error)=w944) -> (error out=w960:errorcluster)  [unwired: 1 in, 2 out]
        n275 = Merge Errors(w961, w960, w951, w950, w949) -> (w962:errorcluster)
      }
    }
    n276 = Or(x="stop", y=w21) -> (x .or. y?=w22:bool)
    "Enum" <- w9
  }
  "error IO" <- w6
